vi "SetSomeDataByLabVIEW.vi"() -> ()   [LabVIEW 2020]
panel:
  out "SLM_NewPulseParameters":cluster{"Freq":i32, "PulseMode":u8}
  out "SOMD_Sync":bool
  out "SOMD_NewBurstValues":T1
  out "VIR_NewFanRunning":bool
  out "VUV_NewFanRunning":bool
  out "VIR_NewIntensity":i32
  out "VUV_NewIntensity":i32
  out "VIR_NewFreqDivIdx":i32
  out "VUV_NewFreqDivIdx":i32
  out "VIR_NewTrigSrcIdx":i32
  out "VUV_NewTrigSrcIdx":i32
  out "VUV_NewTriggerLevel":i32
  out "VIR_NewTriggerLevel":i32
  out "IsVIRModule":bool
  out "VUV_VIR_ModuleType":i32
  out "SOM_NewBurstLengthArray":i32[](array[numeric])
  out "SOM_NewOutNSyncEnable":T2 {"OutEnable" format="%08b"; "SyncEnable" format="%08b"}
  out "SOM_NewBurstValues":T3
  out "SOM_NewFreqTrigMode":i32
  out "SLM_NewIntensity":u16
  out "PRI_NewIntensity":u16
  out "PRI_NewWLIdx":i32
  out "PRI_NewOpModeIdx":i32
  out "Lib Version":string
  out "ModTypAbbr":T4
  out "IsSOMDModule":bool
  out "SOM_ModuleType":i32
  out "PRIConst":T5={"bInitialized"=FALSE, "PrimaModuleID"="", "PrimaModuleType"="", "PrimaFWVers"="", "PrimaTemp_min"=15.0, "PrimaTemp_max"=42.0, "PrimaUSBIdx"=-1, "PrimaSlotId"=-1, "PrimaWLCount"=-1, "PrimaWLs"=[0, 0, 0, -1, -1, -1], "PrimaOpModCount"=-1, "PrimaOpModOff"=-1, "PrimaOpModNarrow"=-1, "PrimaOpModBroad"=-1, "PrimaOpModCW"=-1, "PrimaTrSrcCount"=-1, "PrimaTrSrcInt"=-1, "PrimaTrSrcExtNIM"=-1, "PrimaTrSrcExtTTL"=-1, "PrimaTrSrcExtFallling"=-1, "PrimaTrSrcExtRising"=-1} {"PrimaTemp_min" format="%4.1f"; "PrimaTemp_max" format="%4.1f"; "PrimaSlotId" format="%03d"}
  out "SlotNrsFound":T6 {"SOMSlot" format="%03d"; "SLMSlot" format="%03d"; "VUVSlot" format="%03d"; "VIRSlot" format="%03d"; "PRISlot" format="%03d"}
  out "SerNrsFound":T7
  out "ModTypFound":T8
  out "FW Version":string
  out "clLastFWError":T9
  out "cLastErrorPhase":string
  out "cLastErrorText":string
  out "cProductModel":string caption="Product Model"
  out "cDisplay":string
  out "error out":errorcluster
  out "cDescriptor":string caption="Descriptor"
  in  "iPerformRestart":bool caption="Restart"
  out "iModuleCount":i32 caption="Modules"
  out "cSerialNumber":string caption="Serial Number"
  in  "error in (no error)":errorcluster
  in  "iDevIdx":i32 caption="Device Index" min=0 max=7 step=1
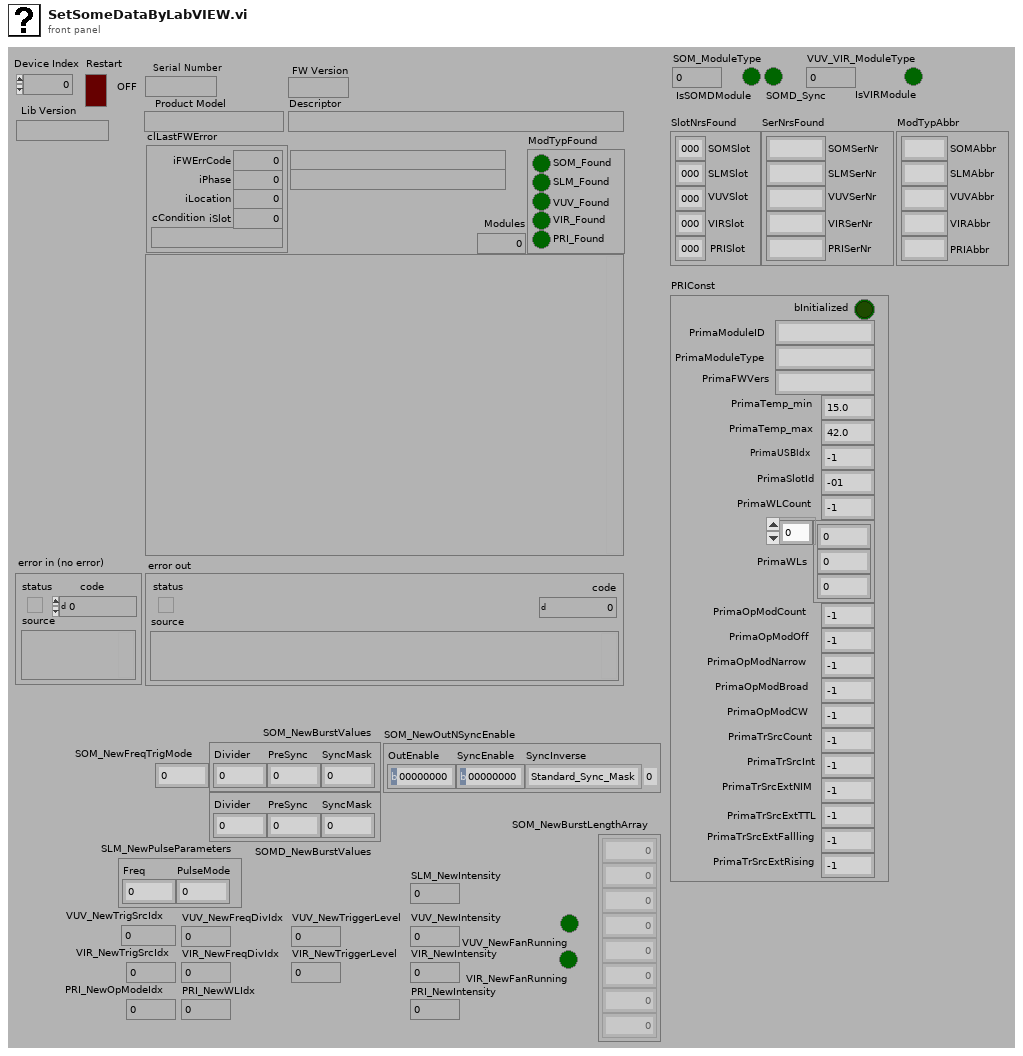
[diagram p1: front panel]
types:
  T1 = cluster{"Divider":u16, "PreSync":u8, "SyncMask":u8}
  T2 = cluster{"OutEnable":u8, "SyncEnable":u8, "SyncInverse":enum8{"Standard_Sync_Mask", "Inverse_Sync_Mask"}}
  T3 = cluster{"Divider":u8, "PreSync":u8, "SyncMask":u8}
  T4 = cluster{"SOMAbbr":string, "SLMAbbr":string, "VUVAbbr":string, "VIRAbbr":string, "PRIAbbr":string}
  T5 = cluster{"bInitialized":bool, "PrimaModuleID":string, "PrimaModuleType":string, "PrimaFWVers":string, "PrimaTemp_min":sgl, "PrimaTemp_max":sgl, "PrimaUSBIdx":i32, "PrimaSlotId":i32, "PrimaWLCount":i32, "PrimaWLs":i32[], "PrimaOpModCount":i32, "PrimaOpModOff":i32, "PrimaOpModNarrow":i32, "PrimaOpModBroad":i32, "PrimaOpModCW":i32, "PrimaTrSrcCount":i32, "PrimaTrSrcInt":i32, "PrimaTrSrcExtNIM":i32, "PrimaTrSrcExtTTL":i32, "PrimaTrSrcExtFallling":i32, "PrimaTrSrcExtRising":i32}
  T6 = cluster{"SOMSlot":i32, "SLMSlot":i32, "VUVSlot":i32, "VIRSlot":i32, "PRISlot":i32}
  T7 = cluster{"SOMSerNr":string, "SLMSerNr":string, "VUVSerNr":string, "VIRSerNr":string, "PRISerNr":string}
  T8 = cluster{"SOM_Found":bool, "SLM_Found":bool, "VUV_Found":bool, "VIR_Found":bool, "PRI_Found":bool}
  T9 = cluster{"iFWErrCode":i32, "iPhase":i32, "iLocation":i32, "iSlot":i32, "cCondition":string}
  T10 = enum16{"open", "replace", "create", "open or create", "replace or create", "replace or create with confirmation"}
  T11 = cluster{"ErrCode":i32, "Error Text":string, "Phase":i32, "Phase Text":string, "Location":i32, "Slot":i32, "Condition":string}
  T12 = cluster{"SlotId":i32, "IsPrimary":u8, "IsBackPlane":u8, "HasUptimeCounter":u8}
  T13 = cluster{"Freq":i32, "PulseMode":u8, "HeadType":i32}
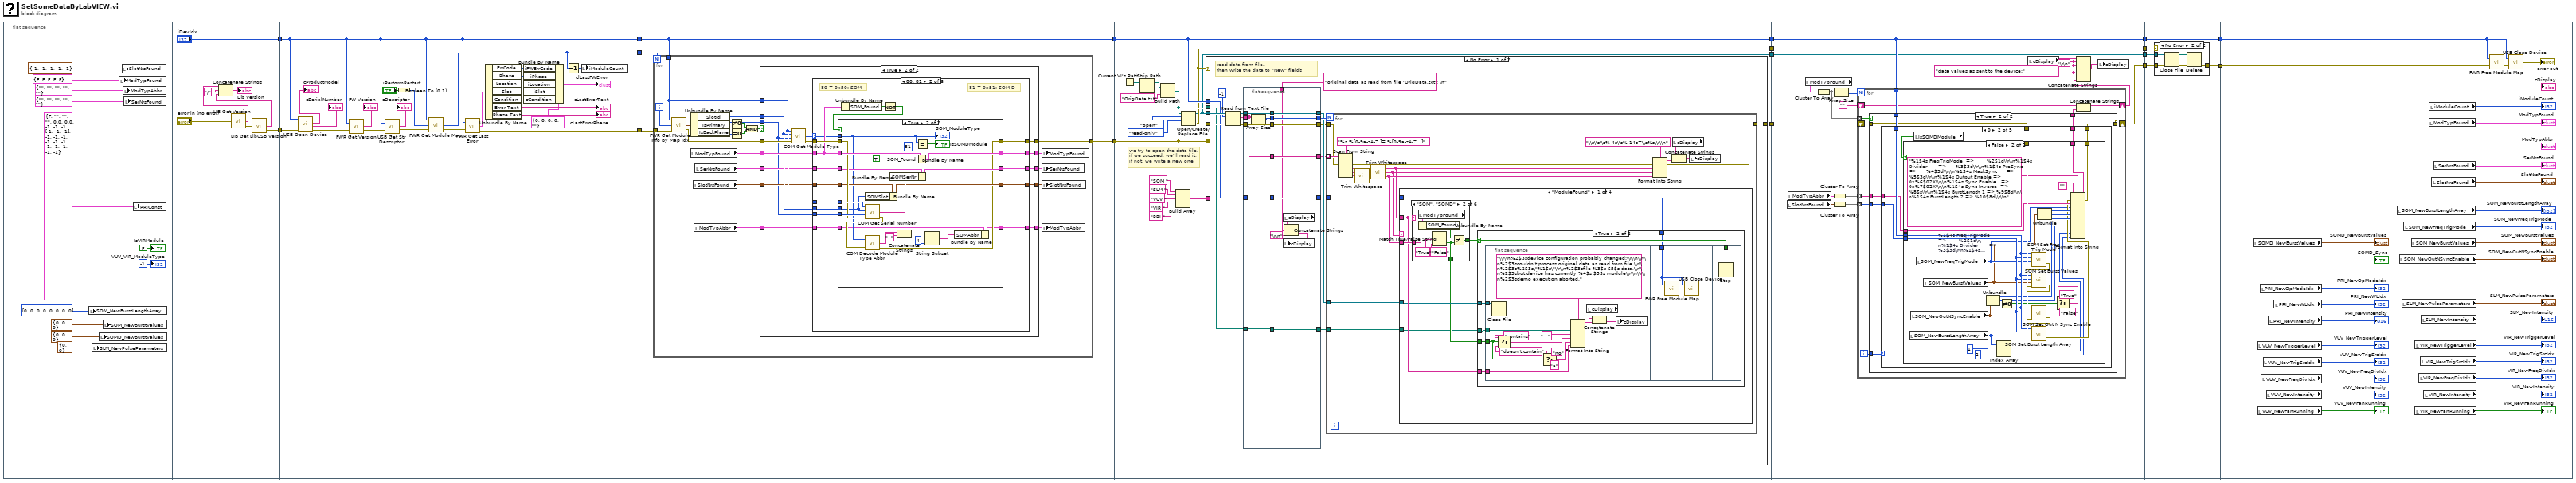
[diagram p0: block diagram]
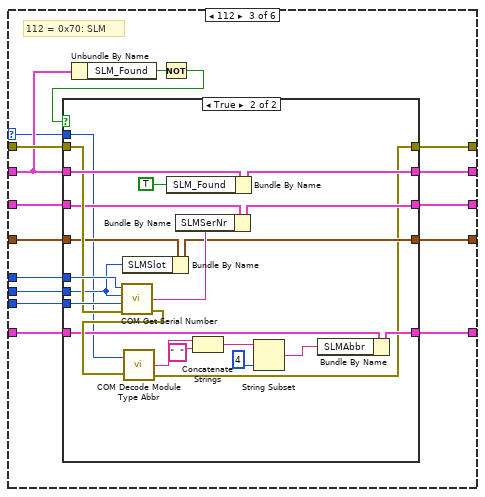
[diagram p5: hidden frame]
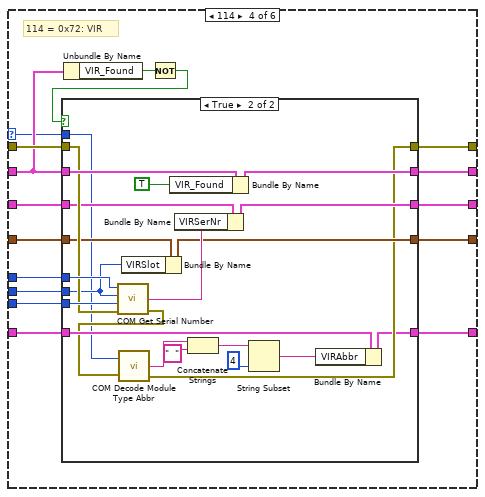
[diagram p7: hidden frame]
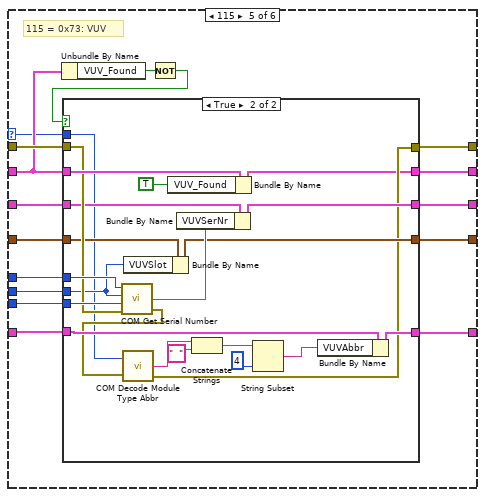
[diagram p9: hidden frame]
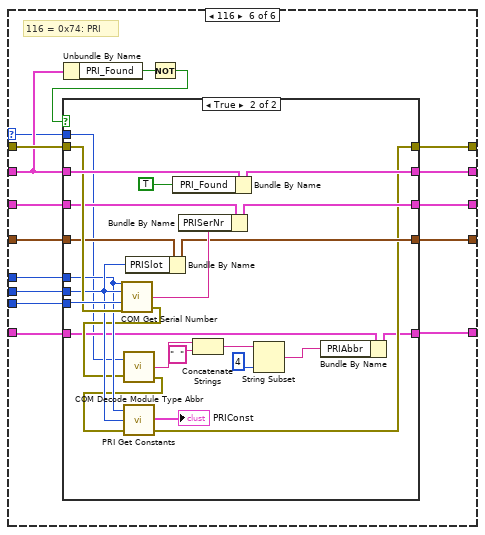
[diagram p11: hidden frame]
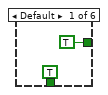
[diagram p14: hidden frame]
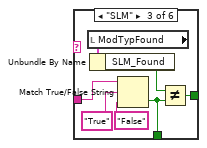
[diagram p15: hidden frame]
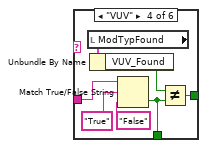
[diagram p16: hidden frame]
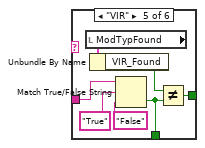
[diagram p17: hidden frame]
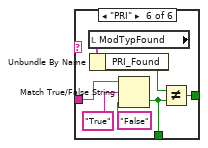
[diagram p18: hidden frame]
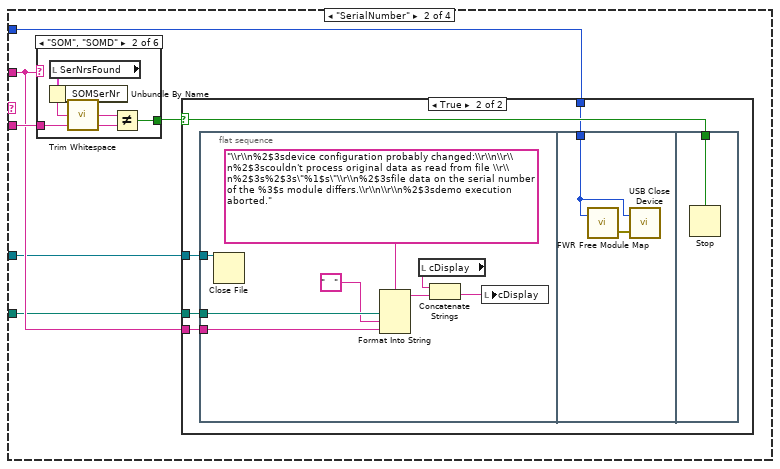
[diagram p19: hidden frame]
diagram:
  n1 = flat-sequence {
    tunnel: ["iDevIdx"] -> w17
    tunnel: [w29] -> w16
    tunnel: w17 -> [w61]
    tunnel: w16 -> [w39]
    tunnel: [w61] -> w15
    tunnel: [w37] -> w14
    tunnel: [w38] -> w13
    tunnel: w15 -> [w62]
    tunnel: w14 -> [w64]
    tunnel: w13 -> [w63]
    tunnel: [w65] -> w12
    tunnel: [w62] -> w11
    tunnel: w12 -> [w334]
    tunnel: w11 -> [w333]
    tunnel: [w333] -> w10
    tunnel: [w332] -> w9
    tunnel: [w331] -> w4
    tunnel: [w330] -> w2
    tunnel: w10 -> [w1031]
    tunnel: w9 -> [w1033]
    tunnel: [w1031] -> w8
    tunnel: [w1032] -> w6
    tunnel: w4 -> [w1027]
    tunnel: [w1027] -> w3
    tunnel: w2 -> [w1026]
    tunnel: [w1026] -> w1
    tunnel: w8 -> [w1206]
    tunnel: [w1206] -> w7
    tunnel: w6 -> [w1203]
    tunnel: [w1202] -> w5
    tunnel: w3 -> [w1205]
    tunnel: w1 -> [w1204]
    tunnel: w7 -> [w1214]
    tunnel: w5 -> [w1213]
    frame #0 {
      n2 = local write "SOM_NewBurstLengthArray"(i32[] [0, 0, 0, 0, 0, 0, 0, 0] ("SOM_NewBurstLengthArray")) -> ()
      n3 = local write "SLM_NewPulseParameters"(cluster{"Freq":i32, "PulseMode":u8} {"Freq"=0, "PulseMode"=0} ("SLM_NewPulseParameters")) -> ()
      n4 = local write "SOMD_NewBurstValues"(T1 {"Divider"=0, "PreSync"=0, "SyncMask"=0} ("SOM_NewBurstValues")) -> ()
      n5 = local write "SOM_NewBurstValues"(T3 {"Divider"=0, "PreSync"=0, "SyncMask"=0} ("SOM_NewBurstValues")) -> ()
      n6 = local write "ModTypFound"(T8 {"SOM_Found"=FALSE, "SLM_Found"=FALSE, "VUV_Found"=FALSE, "VIR_Found"=FALSE, "PRI_Found"=FALSE} ("ModTypFound")) -> ()
      n7 = local write "SlotNrsFound"(T6 {"SOMSlot"=-1, "SLMSlot"=-1, "VUVSlot"=-1, "VIRSlot"=-1, "PRISlot"=-1} ("SlotNrsFound")) -> ()
      n8 = local write "ModTypAbbr"(T4 {"SOMAbbr"="", "SLMAbbr"="", "VUVAbbr"="", "VIRAbbr"="", "PRIAbbr"=""} ("ModTypAbbr")) -> ()
      n9 = local write "SerNrsFound"(T4 {"SOMAbbr"="", "SLMAbbr"="", "VUVAbbr"="", "VIRAbbr"="", "PRIAbbr"=""} ("ModTypAbbr")) -> ()
      n10 = local write "PRIConst"(T5 {"bInitialized"=FALSE, "PrimaModuleID"="", "PrimaModuleType"="", "PrimaFWVers"="", "PrimaTemp_min"=0.0, "PrimaTemp_max"=0.0, "PrimaUSBIdx"=-1, "PrimaSlotId"=-1, "PrimaWLCount"=-1, "PrimaWLs"=[-1, -1, -1], "PrimaOpModCount"=-1, "PrimaOpModOff"=-1, "PrimaOpModNarrow"=-1, "PrimaOpModBroad"=-1, "PrimaOpModCW"=-1, "PrimaTrSrcCount"=-1, "PrimaTrSrcInt"=-1, "PrimaTrSrcExtNIM"=-1, "PrimaTrSrcExtTTL"=-1, "PrimaTrSrcExtFallling"=-1, "PrimaTrSrcExtRising"=-1} ("PRIConst")) -> ()
      "IsVIRModule" <- FALSE ("IsVIRModule")
      "VUV_VIR_ModuleType" <- -1 ("VUV_VIR_ModuleType")
    }
    frame #1 {
      n11 = call "LIB Get Version.vi"("error in (no error)"="error in (no error)") -> ("LibVersion"=w34:string, "error out"=w32:errorcluster)  [unwired: 1 out]
      n12 = call "LIB Get LibUSB Version.vi"("error in (no error)"=w32) -> ("LibUSBVersion"=w33:string, "error out"=w29:errorcluster)  [unwired: 1 out]
      n13 = Concatenate Strings(w34, "/" ("string"), w33) -> (→"Lib Version":string)
    }
    frame #2 {
      n14 = call "USB Open Device.vi"("error in (no error)"=w39, "DevIdx"=w61) -> ("error out"=w57:errorcluster, "SerialNumber"=→"cSerialNumber":string, "ProductModel"=→"cProductModel":string)  [unwired: 2 in, 1 out]
      n15 = call "FWR Get Version.vi"("DevIdx"=w61, "error in (no error)"=w57) -> ("FWVersion"=→"FW Version":string, "error out"=w58:errorcluster)  [unwired: 1 out]
      n16 = call "USB Get Str Descriptor.vi"("DevIdx"=w61, "error in (no error)"=w58) -> ("Descriptor"=→"cDescriptor":string, "error out"=w41:errorcluster)  [unwired: 1 out]
      n17 = Boolean To (0,1)(Boolean="iPerformRestart") -> (0, 1=w55:i16)
      n18 = call "FWR Get Module Map.vi"("error in (no error)"=w41, "PerformRestart"=w55, "DevIdx"=w61) -> ("error out"=w43:errorcluster, "ModuleCount"=w38:i32)  [unwired: 1 out]
      n19 = call "FWR Get Last Error.vi"("DevIdx"=w61, "error in (no error)"=w43) -> ("Last Error"=w54:T11, "error out"=w37:errorcluster)  [unwired: 1 out]
      n20 = Unbundle By Name(w54) -> ("ErrCode"=w46:i32, "Phase"=w47:i32, "Location"=w48:i32, "Slot"=w49:i32, "Condition"=w50:string, "Error Text"=→"cLastErrorText":string, "Phase Text"=→"cLastErrorPhase":string)
      n21 = Bundle By Name(cluster=T9 {"iFWErrCode"=0, "iPhase"=0, "iLocation"=0, "iSlot"=0, "cCondition"=""} ("clLastFWError"), "iFWErrCode"=w46, "iPhase"=w47, "iLocation"=w48, "iSlot"=w49, "cCondition"=w50) -> (→"clLastFWError":T9)
      n22 = Decrement(x=w38) -> (x-1=w60:i32)
      n23 = local write "iModuleCount"(w60) -> ()
    }
    frame #3 {
      n24 = for {
        N: w63 -> [_]
        tunnel: [w75] -> w65
        tunnel: w64 -> [w76]
        tunnel: w62 -> [w78]
        i -> [w84]
        n25 = call "FWR Get Module Info By Map Idx.vi"("error in (no error)"=w76, "MapIdx"=w84, "DevIdx"=w78) -> ("error out"=w74:errorcluster, "FWR Module Info"=w85:T12)  [unwired: 1 out]
        n26 = local read "ModTypFound"() -> (w73:T8)
        n27 = Unbundle By Name(w85) -> ("SlotId"=w79:i32, "IsPrimary"=w77:u8, "IsBackPlane"=w83:u8)
        n28 = local read "SlotNrsFound"() -> (w69:T6)
        n29 = local read "ModTypAbbr"() -> (w67:T4)
        n30 = local read "SerNrsFound"() -> (w71:T7)
        n31 = Not Equal To 0?(x=w77) -> (x != 0?=w81:bool)
        n32 = Equal To 0?(x=w83) -> (x = 0?=w82:bool)
        n33 = And(x=w81, y=w82) -> (x .and. y?=w80:bool)
        n34 = case shown="True" w80 {
          tunnel: w79 -> [_ w98]
          tunnel: w78 -> [_ w99]
          tunnel: w77 -> [_ w91]
          tunnel: w74 -> [w90 w105]
          tunnel: [w90 w103] -> w75
          tunnel: w73 -> [w89 w101]
          tunnel: [w89 w100] -> w72
          tunnel: w71 -> [w88 w97]
          tunnel: [w88 w96] -> w70
          tunnel: w69 -> [w87 w95]
          tunnel: [w87 w94] -> w68
          tunnel: w67 -> [w86 w93]
          tunnel: [w86 w92] -> w66
          frame False {
          }
          frame True {
            n35 = call "COM Get Module Type.vi"("error in (no error)"=w105, "GetPrimary"=w91, "SlotId"=w98, "DevIdx"=w99) -> ("error out"=w104:errorcluster, "ModuleType"=w102:i32)  [unwired: 1 out]
            n36 = case shown="80, 81" w102 {
              selector: w102 -> [_ w113 w156 w199 w242 w285]
              tunnel: w104 -> [w109 w125 w170 w213 w256 w299]
              tunnel: [w109 w124 w169 w212 w255 w298] -> w103
              tunnel: w101 -> [w110 w123 w168 w211 w254 w297]
              tunnel: [w110 w126 w171 w214 w257 w300] -> w100
              tunnel: w99 -> [_ w120 w165 w208 w251 w294]
              tunnel: w98 -> [_ w119 w164 w207 w250 w293]
              tunnel: w91 -> [_ w118 w163 w206 w249 w292]
              tunnel: w97 -> [w108 w117 w162 w205 w248 w291]
              tunnel: [w108 w116 w161 w204 w247 w290] -> w96
              tunnel: w95 -> [w107 w115 w160 w203 w246 w289]
              tunnel: [w107 w114 w159 w202 w245 w288] -> w94
              tunnel: w93 -> [w106 w112 w158 w201 w244 w287]
              tunnel: [w106 w111 w157 w200 w243 w286] -> w92
              frame -1, Default {
              }
              frame 80, 81 {
                # "81 = 0x51: SOM-D"
                # "80 = 0x50: SOM"
                n37 = Unbundle By Name(w123) -> ("SOM_Found"=w122:bool)
                n38 = Not(x=w122) -> (.not. x?=w121:bool)
                n39 = case shown="True" w121 {
                  tunnel: w123 -> [w130 w155]
                  tunnel: [w130 w154] -> w126
                  tunnel: w125 -> [w131 w150]
                  tunnel: [w131 w139] -> w124
                  tunnel: w120 -> [_ w152]
                  tunnel: w119 -> [_ w145]
                  tunnel: w118 -> [_ w151]
                  tunnel: w117 -> [w129 w149]
                  tunnel: [w129 w148] -> w116
                  tunnel: w115 -> [w128 w146]
                  tunnel: [w128 w144] -> w114
                  tunnel: w113 -> [_ w140]
                  tunnel: w112 -> [w127 w138]
                  tunnel: [w127 w137] -> w111
                  frame False {
                  }
                  frame True {
                    n40 = Bundle By Name(cluster=w146, "SOMSlot"=w145) -> (w144:T6)
                    n41 = call "COM Get Serial Number.vi"("error in (no error)"=w150, "GetPrimary"=w151, "SlotId"=w145, "DevIdx"=w152) -> ("error out"=w141:errorcluster, "SerialNumber"=w147:string)  [unwired: 1 out]
                    n42 = call "COM Decode Module Type Abbr.vi"("ModuleType"=w140, "error in (no error)"=w141) -> ("ModulTypeAbbr"=w136:string, "error out"=w139:errorcluster)  [unwired: 1 out]
                    n43 = Bundle By Name(cluster=w155, "SOM_Found"=TRUE ("PRI_Found")) -> (w154:T8)
                    n44 = Bundle By Name(cluster=w149, "SOMSerNr"=w147) -> (w148:T7)
                    n45 = Concatenate Strings(w136, "  ") -> (w134:string)
                    n46 = Equal?(x=w140, y=81) -> (x = y?=→"IsSOMDModule":bool)
                    n47 = String Subset(string=w134, length (rest)=4 ("length (rest)")) -> (substring=w132:string)  [unwired: 1 in]
                    n48 = Bundle By Name(cluster=w138, "SOMAbbr"=w132) -> (w137:T4)
                    "SOM_ModuleType" <- w140
                  }
                }
              }
              frame 112 {
                # "112 = 0x70: SLM"
                n49 = Unbundle By Name(w168) -> ("SLM_Found"=w167:bool)
                n50 = Not(x=w167) -> (.not. x?=w166:bool)
                n51 = case shown="True" w166 {
                  tunnel: w168 -> [w175 w198]
                  tunnel: [w175 w197] -> w171
                  tunnel: w170 -> [w176 w193]
                  tunnel: [w176 w179] -> w169
                  tunnel: w165 -> [_ w195]
                  tunnel: w164 -> [_ w188]
                  tunnel: w163 -> [_ w194]
                  tunnel: w162 -> [w174 w192]
                  tunnel: [w174 w191] -> w161
                  tunnel: w160 -> [w173 w189]
                  tunnel: [w173 w187] -> w159
                  tunnel: w158 -> [w172 w178]
                  tunnel: [w172 w181] -> w157
                  tunnel: w156 -> [_ w177]
                  frame False {
                  }
                  frame True {
                    n52 = call "COM Get Serial Number.vi"("error in (no error)"=w193, "GetPrimary"=w194, "SlotId"=w188, "DevIdx"=w195) -> ("error out"=w180:errorcluster, "SerialNumber"=w190:string)  [unwired: 1 out]
                    n53 = Bundle By Name(cluster=w189, "SLMSlot"=w188) -> (w187:T6)
                    n54 = call "COM Decode Module Type Abbr.vi"("ModuleType"=w177, "error in (no error)"=w180) -> ("ModulTypeAbbr"=w186:string, "error out"=w179:errorcluster)  [unwired: 1 out]
                    n55 = Bundle By Name(cluster=w198, "SLM_Found"=TRUE ("PRI_Found")) -> (w197:T8)
                    n56 = Bundle By Name(cluster=w192, "SLMSerNr"=w190) -> (w191:T7)
                    n57 = Concatenate Strings(w186, "  ") -> (w184:string)
                    n58 = String Subset(string=w184, length (rest)=4 ("length (rest)")) -> (substring=w182:string)  [unwired: 1 in]
                    n59 = Bundle By Name(cluster=w178, "SLMAbbr"=w182) -> (w181:T4)
                  }
                }
              }
              frame 114 {
                # "114 = 0x72: VIR"
                n60 = Unbundle By Name(w211) -> ("VIR_Found"=w210:bool)
                n61 = Not(x=w210) -> (.not. x?=w209:bool)
                n62 = case shown="True" w209 {
                  tunnel: w211 -> [w218 w241]
                  tunnel: [w218 w240] -> w214
                  tunnel: w213 -> [w219 w236]
                  tunnel: [w219 w222] -> w212
                  tunnel: w208 -> [_ w238]
                  tunnel: w207 -> [_ w231]
                  tunnel: w206 -> [_ w237]
                  tunnel: w205 -> [w217 w235]
                  tunnel: [w217 w234] -> w204
                  tunnel: w203 -> [w216 w232]
                  tunnel: [w216 w230] -> w202
                  tunnel: w201 -> [w215 w224]
                  tunnel: [w215 w221] -> w200
                  tunnel: w199 -> [_ w220]
                  frame False {
                  }
                  frame True {
                    n63 = call "COM Get Serial Number.vi"("error in (no error)"=w236, "GetPrimary"=w237, "SlotId"=w231, "DevIdx"=w238) -> ("error out"=w223:errorcluster, "SerialNumber"=w233:string)  [unwired: 1 out]
                    n64 = call "COM Decode Module Type Abbr.vi"("ModuleType"=w220, "error in (no error)"=w223) -> ("ModulTypeAbbr"=w229:string, "error out"=w222:errorcluster)  [unwired: 1 out]
                    n65 = Bundle By Name(cluster=w232, "VIRSlot"=w231) -> (w230:T6)
                    n66 = Bundle By Name(cluster=w241, "VIR_Found"=TRUE ("PRI_Found")) -> (w240:T8)
                    n67 = Bundle By Name(cluster=w235, "VIRSerNr"=w233) -> (w234:T7)
                    n68 = Concatenate Strings(w229, "  ") -> (w227:string)
                    n69 = String Subset(string=w227, length (rest)=4 ("length (rest)")) -> (substring=w225:string)  [unwired: 1 in]
                    n70 = Bundle By Name(cluster=w224, "VIRAbbr"=w225) -> (w221:T4)
                  }
                }
              }
              frame 115 {
                # "115 = 0x73: VUV"
                n71 = Unbundle By Name(w254) -> ("VUV_Found"=w253:bool)
                n72 = Not(x=w253) -> (.not. x?=w252:bool)
                n73 = case shown="True" w252 {
                  tunnel: w254 -> [w261 w284]
                  tunnel: [w261 w263] -> w257
                  tunnel: w256 -> [w262 w280]
                  tunnel: [w262 w265] -> w255
                  tunnel: w251 -> [_ w282]
                  tunnel: w250 -> [_ w275]
                  tunnel: w249 -> [_ w281]
                  tunnel: w248 -> [w260 w279]
                  tunnel: [w260 w278] -> w247
                  tunnel: w246 -> [w259 w276]
                  tunnel: [w259 w274] -> w245
                  tunnel: w244 -> [w258 w268]
                  tunnel: [w258 w267] -> w243
                  tunnel: w242 -> [_ w264]
                  frame False {
                  }
                  frame True {
                    n74 = call "COM Get Serial Number.vi"("error in (no error)"=w280, "GetPrimary"=w281, "SlotId"=w275, "DevIdx"=w282) -> ("error out"=w266:errorcluster, "SerialNumber"=w277:string)  [unwired: 1 out]
                    n75 = call "COM Decode Module Type Abbr.vi"("ModuleType"=w264, "error in (no error)"=w266) -> ("ModulTypeAbbr"=w273:string, "error out"=w265:errorcluster)  [unwired: 1 out]
                    n76 = Bundle By Name(cluster=w276, "VUVSlot"=w275) -> (w274:T6)
                    n77 = Bundle By Name(cluster=w284, "VUV_Found"=TRUE ("PRI_Found")) -> (w263:T8)
                    n78 = Bundle By Name(cluster=w279, "VUVSerNr"=w277) -> (w278:T7)
                    n79 = Concatenate Strings(w273, "  ") -> (w271:string)
                    n80 = String Subset(string=w271, length (rest)=4 ("length (rest)")) -> (substring=w269:string)  [unwired: 1 in]
                    n81 = Bundle By Name(cluster=w268, "VUVAbbr"=w269) -> (w267:T4)
                  }
                }
              }
              frame 116 {
                # "116 = 0x74: PRI"
                n82 = Unbundle By Name(w297) -> ("PRI_Found"=w296:bool)
                n83 = Not(x=w296) -> (.not. x?=w295:bool)
                n84 = case shown="True" w295 {
                  tunnel: w297 -> [w304 w329]
                  tunnel: [w304 w328] -> w300
                  tunnel: w299 -> [w305 w325]
                  tunnel: [w305 w316] -> w298
                  tunnel: w294 -> [_ w318]
                  tunnel: w293 -> [_ w319]
                  tunnel: w292 -> [_ w326]
                  tunnel: w291 -> [w303 w324]
                  tunnel: [w303 w323] -> w290
                  tunnel: w289 -> [w302 w321]
                  tunnel: [w302 w320] -> w288
                  tunnel: w287 -> [w301 w308]
                  tunnel: [w301 w307] -> w286
                  tunnel: w285 -> [_ w306]
                  frame False {
                  }
                  frame True {
                    n85 = call "COM Get Serial Number.vi"("error in (no error)"=w325, "GetPrimary"=w326, "SlotId"=w319, "DevIdx"=w318) -> ("error out"=w310:errorcluster, "SerialNumber"=w322:string)  [unwired: 1 out]
                    n86 = call "COM Decode Module Type Abbr.vi"("ModuleType"=w306, "error in (no error)"=w310) -> ("ModulTypeAbbr"=w315:string, "error out"=w309:errorcluster)  [unwired: 1 out]
                    n87 = call "PRI Get Constants.vi"("error in (no error)"=w309, "SlotId"=w319, "DevIdx"=w318) -> ("error out"=w316:errorcluster, "PRIConst"=→"PRIConst":T5)  [unwired: 1 out]
                    n88 = Bundle By Name(cluster=w321, "PRISlot"=w319) -> (w320:T6)
                    n89 = Bundle By Name(cluster=w329, "PRI_Found"=TRUE) -> (w328:T8)
                    n90 = Bundle By Name(cluster=w324, "PRISerNr"=w322) -> (w323:T7)
                    n91 = Concatenate Strings(w315, "  ") -> (w313:string)
                    n92 = String Subset(string=w313, length (rest)=4 ("length (rest)")) -> (substring=w311:string)  [unwired: 1 in]
                    n93 = Bundle By Name(cluster=w308, "PRIAbbr"=w311) -> (w307:T4)
                  }
                }
              }
            }
          }
        }
        n94 = local write "ModTypFound"(w72) -> ()
        n95 = local write "SerNrsFound"(w70) -> ()
        n96 = local write "SlotNrsFound"(w68) -> ()
        n97 = local write "ModTypAbbr"(w66) -> ()
      }
    }
    frame #4 {
      # "we try to open the data file.\nif we succeed, we'll read it,\nif not, we write a new one"
      n98 = Current VI's Path() -> (path=w344:path)
      n99 = Strip Path(path=w344) -> (stripped path=w343:path)  [unwired: 1 out]
      n100 = Build Path(base path=w343, name or relative path="OrigData.txt") -> (appended path=w345:path)
      n101 = Build Array("SOM " ("element"), "SLM " ("element"), "VUV " ("element"), "VIR " ("element"), "PRI " ("element")) -> (w346:string[])
      n102 = Open/Create/Replace File(file path (use dialog)=w345, error in=w334, operation (0:open)=T10."open", access (0:read/write)=enum16{"read/write", "read-only", "write-only"}."read-only") -> (refnum out=w330:refnum<file>, error out=w331:errorcluster)  [unwired: 2 in, 1 out]
      n103 = case shown="No Error" w331 {
        tunnel: w330 -> [w368 _]
        tunnel: w345 -> [w355 w756]
        tunnel: w333 -> [w357 w755]
        tunnel: w334 -> [_ w757]
        tunnel: [w364 w752] -> w332
        tunnel: w331 -> [w366 w753]
        tunnel: w346 -> [_ w751]
        frame No Error {
          # "read data from file, \nthen write the data to \"New\" fields"
          n104 = Read from Text File(file (use dialog)=w368, count=-1, error in=w366) -> (refnum out=w361:refnum<file>, text=w363:string[], error out=w360:errorcluster)  [unwired: 1 in, 1 out]
          n105 = flat-sequence {
            tunnel: w363 -> [w371]
            tunnel: w361 -> [w373]
            tunnel: w360 -> [w372]
            tunnel: w357 -> [w370]
            tunnel: w355 -> [w369]
            tunnel: [w374] -> w353
            tunnel: [w373] -> w352
            tunnel: [w372] -> w351
            tunnel: [w371] -> w350
            tunnel: [w370] -> w349
            tunnel: [w369] -> w348
            tunnel: [w379] -> w354
            tunnel: [w380] -> w356
            tunnel: [w381] -> w358
            tunnel: [w382] -> w359
            tunnel: [w383] -> w362
            tunnel: [w384] -> w365
            tunnel: w353 -> [w384]
            tunnel: w352 -> [w383]
            tunnel: w351 -> [w382]
            tunnel: w350 -> [w381]
            tunnel: w349 -> [w380]
            tunnel: w348 -> [w379]
            tunnel: "original data as read from file 'OrigData.txt': \n" -> [w376]
            frame #0 {
              n106 = Array Size(array=w371) -> (size(s)=w374:i32)
            }
            frame #1 {
              n107 = local read "cDisplay"() -> (w377:string)
              n108 = Concatenate Strings(w377, w376, "\r\n") -> (w378:string)
              n109 = local write "cDisplay"(w378) -> ()
            }
          }
          n110 = for {
            N: w365 -> [_]
            tunnel: [w385] -> w364
            tunnel: w359 -> [w387]
            tunnel: w358 -> [w401] mode=indexing
            tunnel: w362 -> [w390]
            tunnel: w354 -> [w389]
            tunnel: w356 -> [w388]
            n111 = Scan From String(format string="%s %[0-9a-zA-Z ]= %[0-9a-zA-Z., ]", input string=w401, error in=w387) -> (error out=w386:errorcluster, output 1=w394:string, output 2=w395:string, output 3=w393:string)  [unwired: 4 in, 2 out]
            n112 = call <vilib>:"Trim Whitespace.vi"("string"=w393) -> ("trimmed string"=w392:string)  [unwired: 1 in]
            n113 = call <vilib>:"Trim Whitespace.vi"("string"=w395) -> ("trimmed string"=w391:string)  [unwired: 1 in]
            n114 = case shown="\"ModuleFound\"" w391 {
              selector: w391 -> [_ _ _ w567]
              tunnel: w394 -> [w406 w474 w521 w568]
              tunnel: w392 -> [w408 w475 w523 w566]
              tunnel: w390 -> [w405 w472 w520 _]
              tunnel: w389 -> [w402 w473 w519 _]
              tunnel: w388 -> [w403 w471 w518 _]
              frame "ModuleFound" {
                n115 = case shown="\"SOM\", \"SOMD\"" w406 {
                  tunnel: w408 -> [_ w439 w446 w453 w460 w467]
                  tunnel: [TRUE w436 w443 w450 w457 w464] -> w407
                  tunnel: [TRUE ("selection") w435 w442 w449 w456 w463] -> w404
                  frame Default {
                  }
                  frame "SOM", "SOMD" {
                    n116 = local read "ModTypFound"() -> (w441:T8)
                    n117 = Unbundle By Name(w441) -> ("SOM_Found"=w440:bool)
                    n118 = Match True/False String(2:"False", 3:"True", 4:w439) -> (0:w435:bool)  [unwired: 1 out]
                    n119 = Not Equal?(x=w440, y=w435) -> (x != y?=w436:bool)
                  }
                  frame "SLM" {
                    n120 = local read "ModTypFound"() -> (w448:T8)
                    n121 = Unbundle By Name(w448) -> ("SLM_Found"=w447:bool)
                    n122 = Match True/False String(2:"False", 3:"True", 4:w446) -> (0:w442:bool)  [unwired: 1 out]
                    n123 = Not Equal?(x=w447, y=w442) -> (x != y?=w443:bool)
                  }
                  frame "VUV" {
                    n124 = local read "ModTypFound"() -> (w455:T8)
                    n125 = Unbundle By Name(w455) -> ("VUV_Found"=w454:bool)
                    n126 = Match True/False String(2:"False", 3:"True", 4:w453) -> (0:w449:bool)  [unwired: 1 out]
                    n127 = Not Equal?(x=w454, y=w449) -> (x != y?=w450:bool)
                  }
                  frame "VIR" {
                    n128 = local read "ModTypFound"() -> (w462:T8)
                    n129 = Unbundle By Name(w462) -> ("VIR_Found"=w461:bool)
                    n130 = Match True/False String(2:"False", 3:"True", 4:w460) -> (0:w456:bool)  [unwired: 1 out]
                    n131 = Not Equal?(x=w461, y=w456) -> (x != y?=w457:bool)
                  }
                  frame "PRI" {
                    n132 = local read "ModTypFound"() -> (w469:T8)
                    n133 = Unbundle By Name(w469) -> ("PRI_Found"=w468:bool)
                    n134 = Match True/False String(2:"False", 3:"True", 4:w467) -> (0:w463:bool)  [unwired: 1 out]
                    n135 = Not Equal?(x=w468, y=w463) -> (x != y?=w464:bool)
                  }
                }
                n136 = case shown="True" w407 {
                  selector: w407 -> [_ w413]
                  tunnel: w405 -> [_ w414]
                  tunnel: w404 -> [_ w412]
                  tunnel: w402 -> [_ w411]
                  tunnel: w403 -> [_ w410]
                  tunnel: w406 -> [_ w409]
                  frame False {
                  }
                  frame True {
                    n137 = flat-sequence {
                      tunnel: w414 -> [w427]
                      tunnel: w412 -> [w421]
                      tunnel: w411 -> [w424]
                      tunnel: w409 -> [w415]
                      tunnel: w410 -> [w431]
                      tunnel: w413 -> [w432]
                      frame #0 {
                        n138 = Close File(refnum=w427) -> ()  [unwired: 1 in, 2 out]
                        n139 = Select(t="contains", s=w421, f="doesn't contain") -> (s? t:f=w417:string)
                        n140 = Select(t="no", s=w421, f="a") -> (s? t:f=w418:string)
                        n141 = Format Into String(format string="\\r\\n%2$3sdevice configuration probably changed:\\r\\n\\r\\n%2$3scouldn't process original data as read from file \\r\\n%2$3s%2$3s\"%1$s\"\\r\\n%2$3sfile %3$s $5$s data,\\r\\n%2$3sbut device has currently %4$s $5$s module\\r\\n\\r\\n%2$3sdemo execution aborted." ("string"), w424, "   " ("input 2"), w417, w418, w415) -> (resulting string=w426:string)  [unwired: 2 in, 1 out]
                        n142 = local read "cDisplay"() -> (w428:string)
                        n143 = Concatenate Strings(w428, w426) -> (w429:string)
                        n144 = local write "cDisplay"(w429) -> ()
                      }
                      frame #1 {
                        n145 = call "FWR Free Module Map.vi"("DevIdx"=w431) -> ("error out"=w430:errorcluster)  [unwired: 1 in, 1 out]
                        n146 = call "USB Close Device.vi"("error in (no error)"=w430, "DevIdx"=w431) -> ()  [unwired: 1 out]
                      }
                      frame #2 {
                        n147 = Stop(stop? (T)=w432) -> ()
                      }
                    }
                  }
                }
              }
              frame "SerialNumber" {
                n148 = case shown="\"SOM\", \"SOMD\"" w474 {
                  tunnel: w475 -> [_ w496 w501 w506 w511 w516]
                  tunnel: [TRUE w493 w498 w503 w508 w513] -> w470
                  frame Default {
                  }
                  frame "SOM", "SOMD" {
                    n149 = local read "SerNrsFound"() -> (w497:T7)
                    n150 = Unbundle By Name(w497) -> ("SOMSerNr"=w495:string)
                    n151 = call <vilib>:"Trim Whitespace.vi"("string"=w495) -> ("trimmed string"=w494:string)  [unwired: 1 in]
                    n152 = Not Equal?(x=w494, y=w496) -> (x != y?=w493:bool)
                  }
                  frame "SLM" {
                    n153 = local read "SerNrsFound"() -> (w502:T7)
                    n154 = Unbundle By Name(w502) -> ("SLMSerNr"=w500:string)
                    n155 = call <vilib>:"Trim Whitespace.vi"("string"=w500) -> ("trimmed string"=w499:string)  [unwired: 1 in]
                    n156 = Not Equal?(x=w499, y=w501) -> (x != y?=w498:bool)
                  }
                  frame "VUV" {
                    n157 = local read "SerNrsFound"() -> (w507:T7)
                    n158 = Unbundle By Name(w507) -> ("VUVSerNr"=w505:string)
                    n159 = call <vilib>:"Trim Whitespace.vi"("string"=w505) -> ("trimmed string"=w504:string)  [unwired: 1 in]
                    n160 = Not Equal?(x=w504, y=w506) -> (x != y?=w503:bool)
                  }
                  frame "VIR" {
                    n161 = local read "SerNrsFound"() -> (w512:T7)
                    n162 = Unbundle By Name(w512) -> ("VIRSerNr"=w510:string)
                    n163 = call <vilib>:"Trim Whitespace.vi"("string"=w510) -> ("trimmed string"=w509:string)  [unwired: 1 in]
                    n164 = Not Equal?(x=w509, y=w511) -> (x != y?=w508:bool)
                  }
                  frame "PRI" {
                    n165 = local read "SerNrsFound"() -> (w517:T7)
                    n166 = Unbundle By Name(w517) -> ("PRISerNr"=w515:string)
                    n167 = call <vilib>:"Trim Whitespace.vi"("string"=w515) -> ("trimmed string"=w514:string)  [unwired: 1 in]
                    n168 = Not Equal?(x=w514, y=w516) -> (x != y?=w513:bool)
                  }
                }
                n169 = case shown="True" w470 {
                  selector: w470 -> [_ w479]
                  tunnel: w472 -> [_ w480]
                  tunnel: w473 -> [_ w478]
                  tunnel: w471 -> [_ w477]
                  tunnel: w474 -> [_ w476]
                  frame False {
                  }
                  frame True {
                    n170 = flat-sequence {
                      tunnel: w480 -> [w486]
                      tunnel: w478 -> [w483]
                      tunnel: w476 -> [w481]
                      tunnel: w477 -> [w490]
                      tunnel: w479 -> [w491]
                      frame #0 {
                        n171 = Close File(refnum=w486) -> ()  [unwired: 1 in, 2 out]
                        n172 = Format Into String(format string="\\r\\n%2$3sdevice configuration probably changed:\\r\\n\\r\\n%2$3scouldn't process original data as read from file \\r\\n%2$3s%2$3s\"%1$s\"\\r\\n%2$3sfile data on the serial number of the %3$s module differs.\\r\\n\\r\\n%2$3sdemo execution aborted." ("string"), w483, "   " ("input 2"), w481) -> (resulting string=w485:string)  [unwired: 2 in, 1 out]
                        n173 = local read "cDisplay"() -> (w487:string)
                        n174 = Concatenate Strings(w487, w485) -> (w488:string)
                        n175 = local write "cDisplay"(w488) -> ()
                      }
                      frame #1 {
                        n176 = call "FWR Free Module Map.vi"("DevIdx"=w490) -> ("error out"=w489:errorcluster)  [unwired: 1 in, 1 out]
                        n177 = call "USB Close Device.vi"("error in (no error)"=w489, "DevIdx"=w490) -> ()  [unwired: 1 out]
                      }
                      frame #2 {
                        n178 = Stop(stop? (T)=w491) -> ()
                      }
                    }
                  }
                }
              }
              frame "SlotID" {
                n179 = case shown="\"PRI\"" w521 {
                  tunnel: w523 -> [_ w543 w548 w553 w558 w563]
                  tunnel: [TRUE w541 w546 w551 w556 w561] -> w522
                  frame Default {
                  }
                  frame "SOM", "SOMD" {
                    n180 = local read "SlotNrsFound"() -> (w545:T6)
                    n181 = Unbundle By Name(w545) -> ("SOMSlot"=w544:i32)
                    n182 = Decimal String To Number(string=w543) -> (number=w542:i32)  [unwired: 2 in, 1 out]
                    n183 = Not Equal?(x=w544, y=w542) -> (x != y?=w541:bool)
                  }
                  frame "SLM" {
                    n184 = local read "SlotNrsFound"() -> (w550:T6)
                    n185 = Unbundle By Name(w550) -> ("SLMSlot"=w549:i32)
                    n186 = Decimal String To Number(string=w548) -> (number=w547:i32)  [unwired: 2 in, 1 out]
                    n187 = Not Equal?(x=w549, y=w547) -> (x != y?=w546:bool)
                  }
                  frame "VUV" {
                    n188 = local read "SlotNrsFound"() -> (w555:T6)
                    n189 = Unbundle By Name(w555) -> ("VUVSlot"=w554:i32)
                    n190 = Decimal String To Number(string=w553) -> (number=w552:i32)  [unwired: 2 in, 1 out]
                    n191 = Not Equal?(x=w554, y=w552) -> (x != y?=w551:bool)
                  }
                  frame "VIR" {
                    n192 = local read "SlotNrsFound"() -> (w560:T6)
                    n193 = Unbundle By Name(w560) -> ("VIRSlot"=w559:i32)
                    n194 = Decimal String To Number(string=w558) -> (number=w557:i32)  [unwired: 2 in, 1 out]
                    n195 = Not Equal?(x=w559, y=w557) -> (x != y?=w556:bool)
                  }
                  frame "PRI" {
                    n196 = local read "SlotNrsFound"() -> (w565:T6)
                    n197 = Unbundle By Name(w565) -> ("PRISlot"=w564:i32)
                    n198 = Decimal String To Number(string=w563) -> (number=w562:i32)  [unwired: 2 in, 1 out]
                    n199 = Not Equal?(x=w564, y=w562) -> (x != y?=w561:bool)
                  }
                }
                n200 = case shown="True" w522 {
                  selector: w522 -> [_ w527]
                  tunnel: w520 -> [_ w528]
                  tunnel: w519 -> [_ w526]
                  tunnel: w518 -> [_ w525]
                  tunnel: w521 -> [_ w524]
                  tunnel: w522 -> [_ _]
                  frame False {
                  }
                  frame True {
                    n201 = flat-sequence {
                      tunnel: w528 -> [w534]
                      tunnel: w526 -> [w531]
                      tunnel: w524 -> [w529]
                      tunnel: w525 -> [w538]
                      tunnel: w527 -> [w539]
                      frame #0 {
                        n202 = Close File(refnum=w534) -> ()  [unwired: 1 in, 2 out]
                        n203 = Format Into String(format string="\\r\\n%2$3sdevice configuration probably changed:\\r\\n\\r\\n%2$3scouldn't process original data as read from file \\r\\n%2$3s%2$3s\"%1$s\"\\r\\n%2$3sfile data on the slot number of the %3$s module differs.\\r\\n\\r\\n%2$3sdemo execution aborted." ("string"), w531, "   " ("input 2"), w529) -> (resulting string=w533:string)  [unwired: 2 in, 1 out]
                        n204 = local read "cDisplay"() -> (w535:string)
                        n205 = Concatenate Strings(w535, w533) -> (w536:string)
                        n206 = local write "cDisplay"(w536) -> ()
                      }
                      frame #1 {
                        n207 = call "FWR Free Module Map.vi"("DevIdx"=w538) -> ("error out"=w537:errorcluster)  [unwired: 1 in, 1 out]
                        n208 = call "USB Close Device.vi"("error in (no error)"=w537, "DevIdx"=w538) -> ()  [unwired: 1 out]
                      }
                      frame #2 {
                        n209 = Stop(stop? (T)=w539) -> ()
                      }
                    }
                  }
                }
              }
              frame Default {
                n210 = case shown="\"VIR\", \"VUV\"" w568 {
                  selector: w568 -> [_ _ _ _ w705 _]
                  tunnel: w567 -> [_ w570 w627 w684 w707 w740]
                  tunnel: w566 -> [_ w569 w626 w683 w706 w739]
                  frame Default {
                  }
                  frame "SOM" {
                    n211 = case shown="\"Divider\", \"MaskSync\", \"PreSync\"" w570 {
                      selector: w570 -> [_ w576 w594 w620 _]
                      tunnel: w569 -> [w572 w575 w593 w619 _]
                      frame "FreqTrigMode" {
                        n212 = Decimal String To Number(string=w572) -> (number=w571:i32)  [unwired: 2 in, 1 out]
                        n213 = local write "SOM_NewFreqTrigMode"(w571) -> ()
                      }
                      frame "Divider", "MaskSync", "PreSync" {
                        n214 = local read "SOM_NewBurstValues"() -> (w573:T3)
                        n215 = case shown="\"Divider\"" w576 {
                          tunnel: w575 -> [_ w582 w587 w592]
                          tunnel: [w577 w581 w586 w591] -> w574
                          tunnel: w573 -> [w577 w580 w585 w590]
                          frame Default {
                          }
                          frame "Divider" {
                            n216 = Decimal String To Number(string=w582, default (0L)=u8 0 ("default (0 I32)")) -> (number=w579:u8)  [unwired: 1 in, 1 out]
                            n217 = Bundle By Name(cluster=w580, "Divider"=w579) -> (w581:T3)
                          }
                          frame "PreSync" {
                            n218 = Decimal String To Number(string=w587, default (0L)=u8 0 ("default (0 I32)")) -> (number=w584:u8)  [unwired: 1 in, 1 out]
                            n219 = Bundle By Name(cluster=w585, "PreSync"=w584) -> (w586:T3)
                          }
                          frame "MaskSync" {
                            n220 = Decimal String To Number(string=w592, default (0L)=u8 0 ("default (0 I32)")) -> (number=w589:u8)  [unwired: 1 in, 1 out]
                            n221 = Bundle By Name(cluster=w590, "SyncMask"=w589) -> (w591:T3)
                          }
                        }
                        n222 = local write "SOM_NewBurstValues"(w574) -> ()
                      }
                      frame "Output Enable", "Sync Enable", "Sync Inverse" {
                        n223 = local read "SOM_NewOutNSyncEnable"() -> (w595:T2)
                        n224 = case shown="\"Sync Inverse\"" w594 {
                          tunnel: [w597 w603 w609 w617] -> w596
                          tunnel: w595 -> [w597 w602 w608 w616]
                          tunnel: w593 -> [_ w601 w607 w613]
                          frame Default {
                          }
                          frame "Output Enable" {
                            n225 = Hexadecimal String To Number(string=w601, offset=2, default (0uL)=u8 0 ("default (0 U32)")) -> (number=w598:u8)  [unwired: 1 out]
                            n226 = Bundle By Name(cluster=w602, "OutEnable"=w598) -> (w603:T2)
                          }
                          frame "Sync Enable" {
                            n227 = Hexadecimal String To Number(string=w607, offset=2, default (0uL)=u8 0 ("default (0 U32)")) -> (number=w604:u8)  [unwired: 1 out]
                            n228 = Bundle By Name(cluster=w608, "SyncEnable"=w604) -> (w609:T2)
                          }
                          frame "Sync Inverse" {
                            n229 = Match True/False String(2:"False", 3:"True", 4:w613) -> (0:w612:bool)  [unwired: 1 out]
                            n230 = Boolean To (0,1)(Boolean=w612) -> (0, 1=w611:i16)
                            n231 = To Unsigned Byte Integer(number=w611) -> (unsigned 8bit integer=w610:u8)
                            n232 = Bundle By Name(cluster=w616, "SyncInverse"=w610) -> (w617:T2)
                          }
                        }
                        n233 = local write "SOM_NewOutNSyncEnable"(w596) -> ()
                      }
                      frame "BurstLength 1".."BurstLength 9" {
                        n234 = Decimal String To Number(string=w619) -> (number=w618:i32)  [unwired: 2 in, 1 out]
                        n235 = Scan From String(format string="BurstLength %1d", input string=w620) -> (output 1=w624:i32)  [unwired: 3 in, 3 out]
                        n236 = Decrement(x=w624) -> (x-1=w623:i32)
                        n237 = local read "SOM_NewBurstLengthArray"() -> (w622:i32[])
                        n238 = Replace Array Subset(array=w622, new element=w618, index=w623) -> (w621:i32[])
                        n239 = local write "SOM_NewBurstLengthArray"(w621) -> ()
                      }
                      frame Default {
                      }
                    }
                  }
                  frame "SOMD" {
                    n240 = case shown="\"Divider\", \"MaskSync\", \"PreSync\"" w627 {
                      selector: w627 -> [_ w633 w651 w677 _]
                      tunnel: w626 -> [w629 w632 w650 w676 _]
                      frame "FreqTrigMode" {
                        n241 = Decimal String To Number(string=w629) -> (number=w628:i32)  [unwired: 2 in, 1 out]
                        n242 = local write "SOM_NewFreqTrigMode"(w628) -> ()
                      }
                      frame "Divider", "MaskSync", "PreSync" {
                        n243 = local read "SOMD_NewBurstValues"() -> (w630:T1)
                        n244 = case shown="\"MaskSync\"" w633 {
                          tunnel: w632 -> [_ w639 w644 w649]
                          tunnel: [w634 w638 w643 w648] -> w631
                          tunnel: w630 -> [w634 w637 w642 w647]
                          frame Default {
                          }
                          frame "Divider" {
                            n245 = Decimal String To Number(string=w639, default (0L)=u16 0 ("default (0 I32)")) -> (number=w636:u16)  [unwired: 1 in, 1 out]
                            n246 = Bundle By Name(cluster=w637, "Divider"=w636) -> (w638:T1)
                          }
                          frame "PreSync" {
                            n247 = Decimal String To Number(string=w644, default (0L)=u8 0 ("default (0 I32)")) -> (number=w641:u8)  [unwired: 1 in, 1 out]
                            n248 = Bundle By Name(cluster=w642, "PreSync"=w641) -> (w643:T1)
                          }
                          frame "MaskSync" {
                            n249 = Decimal String To Number(string=w649, default (0L)=u8 0 ("default (0 I32)")) -> (number=w646:u8)  [unwired: 1 in, 1 out]
                            n250 = Bundle By Name(cluster=w647, "SyncMask"=w646) -> (w648:T1)
                          }
                        }
                        n251 = local write "SOMD_NewBurstValues"(w631) -> ()
                      }
                      frame "Output Enable", "Sync Enable", "Sync Inverse" {
                        n252 = local read "SOM_NewOutNSyncEnable"() -> (w652:T2)
                        n253 = case shown="\"Sync Inverse\"" w651 {
                          tunnel: [w654 w660 w666 w674] -> w653
                          tunnel: w652 -> [w654 w659 w665 w673]
                          tunnel: w650 -> [_ w658 w664 w670]
                          frame Default {
                          }
                          frame "Output Enable" {
                            n254 = Hexadecimal String To Number(string=w658, offset=2, default (0uL)=u8 0 ("default (0 U32)")) -> (number=w655:u8)  [unwired: 1 out]
                            n255 = Bundle By Name(cluster=w659, "OutEnable"=w655) -> (w660:T2)
                          }
                          frame "Sync Enable" {
                            n256 = Hexadecimal String To Number(string=w664, offset=2, default (0uL)=u8 0 ("default (0 U32)")) -> (number=w661:u8)  [unwired: 1 out]
                            n257 = Bundle By Name(cluster=w665, "SyncEnable"=w661) -> (w666:T2)
                          }
                          frame "Sync Inverse" {
                            n258 = Match True/False String(2:"False", 3:"True", 4:w670) -> (0:w669:bool)  [unwired: 1 out]
                            n259 = Boolean To (0,1)(Boolean=w669) -> (0, 1=w668:i16)
                            n260 = To Unsigned Byte Integer(number=w668) -> (unsigned 8bit integer=w667:u8)
                            n261 = Bundle By Name(cluster=w673, "SyncInverse"=w667) -> (w674:T2)
                          }
                        }
                        n262 = local write "SOM_NewOutNSyncEnable"(w653) -> ()
                      }
                      frame "BurstLength 1".."BurstLength 9" {
                        n263 = Decimal String To Number(string=w676) -> (number=w675:i32)  [unwired: 2 in, 1 out]
                        n264 = Scan From String(format string="BurstLength %1d", input string=w677) -> (output 1=w681:i32)  [unwired: 3 in, 3 out]
                        n265 = Decrement(x=w681) -> (x-1=w680:i32)
                        n266 = local read "SOM_NewBurstLengthArray"() -> (w679:i32[])
                        n267 = Replace Array Subset(array=w679, new element=w675, index=w680) -> (w678:i32[])
                        n268 = local write "SOM_NewBurstLengthArray"(w678) -> ()
                      }
                      frame Default {
                      }
                    }
                  }
                  frame "SLM" {
                    n269 = case shown="\"FreqTrigIdx\"" w684 {
                      tunnel: w683 -> [_ w688 w693 w702]
                      frame Default {
                      }
                      frame "FreqTrigIdx" {
                        n270 = Decimal String To Number(string=w688) -> (number=w685:i32)  [unwired: 2 in, 1 out]
                        n271 = local read "SLM_NewPulseParameters"() -> (w686:cluster{"Freq":i32, "PulseMode":u8})
                        n272 = Bundle By Name(cluster=w686, "Freq"=w685) -> (w687:cluster{"Freq":i32, "PulseMode":u8})
                        n273 = local write "SLM_NewPulseParameters"(w687) -> ()
                      }
                      frame "Pulse Mode" {
                        n274 = Match True/False String(2:"False", 3:"True", 4:w693) -> (0:w692:bool)  [unwired: 1 out]
                        n275 = Boolean To (0,1)(Boolean=w692) -> (0, 1=w694:i16)
                        n276 = To Unsigned Byte Integer(number=w694) -> (unsigned 8bit integer=w689:u8)
                        n277 = local read "SLM_NewPulseParameters"() -> (w691:cluster{"Freq":i32, "PulseMode":u8})
                        n278 = Bundle By Name(cluster=w691, "PulseMode"=w689) -> (w690:cluster{"Freq":i32, "PulseMode":u8})
                        n279 = local write "SLM_NewPulseParameters"(w690) -> ()
                      }
                      frame "Intensity" {
                        n280 = Fract/Exp String To Number(string=w702, default (0 dbl)=sgl 0.0) -> (number=w699:sgl)  [unwired: 2 in, 1 out]
                        n281 = Multiply(x=u16 10 ("y"), y=w699) -> (x*y=w698:sgl)
                        n282 = To Unsigned Word Integer(number=w698) -> (unsigned 16bit integer=w697:u16)
                        n283 = local write "SLM_NewIntensity"(w697) -> ()
                      }
                    }
                  }
                  frame "VIR", "VUV" {
                    n284 = Equal?(x="VIR", y=w705) -> (x = y?=w703:bool)
                    n285 = case shown="\"FreqDivIdx\"" w707 {
                      tunnel: w706 -> [_ w710 w715 w720 w724 w733]
                      tunnel: w703 -> [_ w708 w713 w718 w729 w736]
                      frame Default {
                      }
                      frame "TrigSrcIdx" {
                        n286 = Decimal String To Number(string=w710) -> (number=w709:i32)  [unwired: 2 in, 1 out]
                        n287 = case shown="True" w708 {
                          tunnel: w709 -> [w711 w712]
                          frame False {
                            n288 = local write "VUV_NewTrigSrcIdx"(w711) -> ()
                          }
                          frame True {
                            n289 = local write "VIR_NewTrigSrcIdx"(w712) -> ()
                          }
                        }
                      }
                      frame "FreqDivIdx" {
                        n290 = Decimal String To Number(string=w715) -> (number=w714:i32)  [unwired: 2 in, 1 out]
                        n291 = case shown="True" w713 {
                          tunnel: w714 -> [w716 w717]
                          frame False {
                            n292 = local write "VUV_NewFreqDivIdx"(w716) -> ()
                          }
                          frame True {
                            n293 = local write "VIR_NewFreqDivIdx"(w717) -> ()
                          }
                        }
                      }
                      frame "TrigLevel" {
                        n294 = Decimal String To Number(string=w720) -> (number=w719:i32)  [unwired: 2 in, 1 out]
                        n295 = case shown="True" w718 {
                          tunnel: w719 -> [w721 w722]
                          frame False {
                            n296 = local write "VUV_NewTriggerLevel"(w721) -> ()
                          }
                          frame True {
                            n297 = local write "VIR_NewTriggerLevel"(w722) -> ()
                          }
                        }
                      }
                      frame "Intensity" {
                        n298 = Fract/Exp String To Number(string=w724, default (0 dbl)=sgl 0.0) -> (number=w726:sgl)  [unwired: 2 in, 1 out]
                        n299 = Multiply(x=u16 10 ("y"), y=w726) -> (x*y=w725:sgl)
                        n300 = To Long Integer(number=w725) -> (32bit integer=w723:i32)
                        n301 = case shown="True" w729 {
                          tunnel: w723 -> [w730 w731]
                          frame False {
                            n302 = local write "VUV_NewIntensity"(w730) -> ()
                          }
                          frame True {
                            n303 = local write "VIR_NewIntensity"(w731) -> ()
                          }
                        }
                      }
                      frame "FanRunning" {
                        n304 = Match True/False String(2:"False", 3:"True", 4:w733) -> (0:w732:bool)  [unwired: 1 out]
                        n305 = case shown="True" w736 {
                          tunnel: w732 -> [w737 w738]
                          frame False {
                            n306 = local write "VUV_NewFanRunning"(w737) -> ()
                          }
                          frame True {
                            n307 = local write "VIR_NewFanRunning"(w738) -> ()
                          }
                        }
                      }
                    }
                    n308 = local write "IsVIRModule"(w703) -> ()
                  }
                  frame "PRI" {
                    n309 = case shown="\"WavelengthIdx\"" w740 {
                      tunnel: w739 -> [_ w742 w744 w746]
                      frame Default {
                      }
                      frame "OperModeIdx" {
                        n310 = Decimal String To Number(string=w742) -> (number=w741:i32)  [unwired: 2 in, 1 out]
                        n311 = local write "PRI_NewOpModeIdx"(w741) -> ()
                      }
                      frame "WavelengthIdx" {
                        n312 = Decimal String To Number(string=w744) -> (number=w743:i32)  [unwired: 2 in, 1 out]
                        n313 = local write "PRI_NewWLIdx"(w743) -> ()
                      }
                      frame "Intensity" {
                        n314 = Fract/Exp String To Number(string=w746, default (0 dbl)=sgl 0.0) -> (number=w748:sgl)  [unwired: 2 in, 1 out]
                        n315 = Multiply(x=u16 10 ("y"), y=w748) -> (x*y=w747:sgl)
                        n316 = To Unsigned Word Integer(number=w747) -> (unsigned 16bit integer=w745:u16)
                        n317 = local write "PRI_NewIntensity"(w745) -> ()
                      }
                    }
                  }
                }
              }
            }
            n318 = Format Into String(format string="\\s\\s\\s%-4s\\s%-14s=\\s%s\\r\\n", error in=w386, w394, w391, w392) -> (resulting string=w397:string, error out=w385:errorcluster)  [unwired: 1 in]
            n319 = local read "cDisplay"() -> (w398:string)
            n320 = Concatenate Strings(w398, w397) -> (w396:string)
            n321 = local write "cDisplay"(w396) -> ()
          }
        }
        frame Error {
          # "save original data in file, modify it,\nthen write data to \"New\" fields"
          n322 = Not Equal?(x=w753, y=w757) -> (x != y?=w754:bool)
          n323 = case shown="True" w754 {
            tunnel: w753 -> [_ w1025]
            tunnel: [w773 w1025] -> w752
            tunnel: w756 -> [w779 _]
            tunnel: w755 -> [w774 _]
            tunnel: w751 -> [w758 _]
            frame True {
              # "write"
              n324 = local read "ModTypFound"() -> (w778:T8)
              n325 = local read "SlotNrsFound"() -> (w776:T6)
              n326 = local read "ModTypAbbr"() -> (w772:T4)
              n327 = local read "SerNrsFound"() -> (w765:T7)
              n328 = Cluster To Array(cluster=w778) -> (array=w766:bool[])
              n329 = Array Size(array=w766) -> (size(s)=w777:i32)
              n330 = Cluster To Array(cluster=w772) -> (array=w771:string[])
              n331 = Cluster To Array(cluster=w765) -> (array=w764:string[])
              n332 = Cluster To Array(cluster=w776) -> (array=w775:i32[])
              n333 = Open/Create/Replace File(file path (use dialog)=w779, error in=errorcluster {"status"=FALSE, "code"=0, "source"=""} ("error in 2 (no error)"), operation (0:open)=T10."create", access (0:read/write)=enum16{"read/write", "read-only", "write-only"}."write-only") -> (refnum out=w770:refnum<file>, error out=w769:errorcluster)  [unwired: 2 in, 1 out]
              n334 = for {
                N: w777 -> [_]
                tunnel: w766 -> [w783] mode=indexing
                tunnel: w775 -> [w794] mode=indexing
                tunnel: w774 -> [w793]
                tunnel: w771 -> [w790] mode=indexing
                tunnel: w769 -> [w792]
                tunnel: [w791] -> w768
                shift-right: [w789] -> w760
                shift-left: "" -> [w784]
                tunnel: w758 -> [w788] mode=indexing
                tunnel: w764 -> [w787] mode=indexing
                i -> [w786]
                n335 = case shown="True" w783 {
                  tunnel: w794 -> [_ w805]
                  tunnel: w793 -> [_ w804]
                  tunnel: w790 -> [_ w803]
                  tunnel: w792 -> [w799 w806]
                  tunnel: [w799 w801] -> w791
                  tunnel: w788 -> [w796 _]
                  tunnel: w787 -> [_ w802]
                  tunnel: w786 -> [_ w807]
                  tunnel: [w795 w800] -> w785
                  frame False {
                    n336 = Format Into String(format string="%1$4s ModuleFound   =        False\\r\\n", initial string="", w796) -> (resulting string=w795:string)  [unwired: 1 in, 1 out]
                  }
                  frame True {
                    n337 = case shown="0" w807 {
                      selector: w807 -> [_ _ _ w977 _]
                      tunnel: w806 -> [w809 w815 w937 w979 w1013]
                      tunnel: [w809 w821 w943 w984 w1014] -> w801
                      tunnel: ["" w818 w942 w983 w1011] -> w800
                      tunnel: w805 -> [_ w812 w934 w955 w1016]
                      tunnel: w804 -> [_ w813 w935 w954 w1019]
                      tunnel: w803 -> [_ w811 w941 w982 w1017]
                      tunnel: w802 -> [_ w820 w940 w981 w1015]
                      frame -1, Default {
                      }
                      frame 0 {
                        n338 = local read "IsSOMDModule"() -> (w817:bool)
                        n339 = case shown="True" w817 {
                          tunnel: [w850 w895] -> w816
                          tunnel: w815 -> [w858 w903]
                          tunnel: [w849 w894] -> w814
                          tunnel: w813 -> [w854 w899]
                          tunnel: w812 -> [w852 w897]
                          tunnel: w811 -> [w832 w877]
                          frame False {
                            w829 = 2
                            w830 = 1
                            w851 = "%1$4s FreqTrigMode  =        %2$1d\\r\\n%1$4s Divider       =      %3$3d\\r\\n%1$4s PreSync       =      %4$3d\\r\\n%1$4s MaskSync      =      %5$3d\\r\\n%1$4s Output Enable =     0x%6$02X\\r\\n%1$4s Sync Enable   =     0x%7$02X\\r\\n%1$4s Sync Inverse  =        %8$s\\r\\n%s"  # %1$4s FreqTrigMode  =        %2$1d\r\n%1$4s Divider       =      %3$3d\r\n%1$4s PreSync       =      %4$3d\r\n%1$4s MaskSync      =      %5$3d\r\n%1$4s Output Enable =     0x%6$02X\r\n%1$4s Sync Enable   =     0x%7$02X\r\n%1$4s Sync Inverse  =        %8$s\r\n%s
                            n340 = call "SOM Get Freq Trig Mode.vi"("error in (no error)"=w858, "SlotId"=w852, "DevIdx"=w854) -> ("error out"=w857:errorcluster, "FreqTrigMode"=w848:i32)  [unwired: 1 out]
                            n341 = call "SOM Get Burst Values.vi"("error in (no error)"=w857, "SlotId"=w852, "DevIdx"=w854) -> ("error out"=w856:errorcluster, "SOM Burst Values"=w847:T3)  [unwired: 1 out]
                            n342 = Unbundle By Name(w847) -> ("Divider"=w846:u8, "PreSync"=w845:u8, "SyncMask"=w844:u8)
                            n343 = call "SOM Get Out N Sync Enable.vi"("error in (no error)"=w856, "SlotId"=w852, "DevIdx"=w854) -> ("error out"=w855:errorcluster, "SOM Out N Sync Enable"=w843:T2)  [unwired: 1 out]
                            n344 = Unbundle By Name(w843) -> ("OutEnable"=w842:u8, "SyncEnable"=w841:u8, "SyncInverse"=w840:enum8{"Standard_Sync_Mask", "Inverse_Sync_Mask"})
                            n345 = Not Equal To 0?(x=w840) -> (x != 0?=w839:bool)
                            n346 = call "SOM Get Burst Length Array.vi"("error in (no error)"=w855, "SlotId"=w852, "DevIdx"=w854) -> ("error out"=w826:errorcluster, "SOM Burst Length Array"=w831:i32[])  [unwired: 1 out]
                            n347 = for {
                              N: 8 -> [_]
                              tunnel: w831 -> [w860] mode=indexing
                              shift-right: [w865] -> w833
                              shift-left: "" -> [w863]
                              tunnel: w832 -> [w862]
                              i -> [w861]
                              n348 = Increment(x=w861) -> (x+1=w859:i32)
                              n349 = Format Into String(format string="%4s BurstLength %d = %8d\\r\\n", initial string=w863, w862, w859, w860) -> (resulting string=w865:string)  [unwired: 1 in, 1 out]
                            }
                            n350 = Index Array(array=w831, index #1=w830, index #2=w829) -> (element #1=w827:i32, element #2=w828:i32)
                            n351 = Select(t="True", s=w839, f="False") -> (s? t:f=w838:string)
                            n352 = Format Into String(format string=w851, initial string="", error in=w826, w832, w848, w846, w845, w844, w842, w841, w838, w833) -> (resulting string=w850:string, error out=w849:errorcluster)
                            n353 = Replace Array Subset(array=w831, new element #1=w828, index #1=w830, new element #2=w827, index #2=w829) -> (w825:i32[])
                            n354 = local write "SOM_NewBurstLengthArray"(w825) -> ()
                            n355 = local write "SOM_NewOutNSyncEnable"(T2 {"OutEnable"=165, "SyncEnable"=147, "SyncInverse"=enum."Inverse_Sync_Mask"} ("SOM_NewOutNSyncEnable")) -> ()
                            n356 = local write "SOM_NewFreqTrigMode"(4 ("SOM_NewFreqTrigMode")) -> ()
                            n357 = local write "SOM_NewBurstValues"(T3 {"Divider"=200, "PreSync"=10, "SyncMask"=1} ("SOM_NewBurstValues")) -> ()
                          }
                          frame True {
                            w875 = 2
                            w876 = 1
                            w896 = "%1$4s FreqTrigMode  =        %2$1d\\r\\n%1$4s Divider       =      %3$3d\\r\\n%1$4s PreSync       =      %4$3d\\r\\n%1$4s MaskSync      =      %5$3d\\r\\n%1$4s Output Enable =     0x%6$02X\\r\\n%1$4s Sync Enable   =     0x%7$02X\\r\\n%1$4s Sync Inverse  =        %8$s\\r\\n%s"  # %1$4s FreqTrigMode  =        %2$1d\r\n%1$4s Divider       =      %3$3d\r\n%1$4s PreSync       =      %4$3d\r\n%1$4s MaskSync      =      %5$3d\r\n%1$4s Output Enable =     0x%6$02X\r\n%1$4s Sync Enable   =     0x%7$02X\r\n%1$4s Sync Inverse  =        %8$s\r\n%s
                            n358 = call "SOMD Get Freq Trig Mode.vi"("DevIdx"=w899, "SlotId"=w897, "error in (no error)"=w903) -> ("FreqTrigMode"=w893:i32, "Synchronize"=w867:bool, "error out"=w902:errorcluster)  [unwired: 1 out]
                            n359 = call "SOMD Get Burst Values.vi"("error in (no error)"=w902, "SlotId"=w897, "DevIdx"=w899) -> ("error out"=w901:errorcluster, "SOMD Burst Values"=w892:T1)  [unwired: 1 out]
                            n360 = Unbundle By Name(w892) -> ("Divider"=w891:u16, "PreSync"=w890:u8, "SyncMask"=w889:u8)
                            n361 = call "SOMD Get Out N Sync Enable.vi"("error in (no error)"=w901, "SlotId"=w897, "DevIdx"=w899) -> ("error out"=w900:errorcluster, "SOMD Out N Sync Enable"=w888:T2)  [unwired: 1 out]
                            n362 = Unbundle By Name(w888) -> ("OutEnable"=w887:u8, "SyncEnable"=w886:u8, "SyncInverse"=w885:enum8{"Standard_Sync_Mask", "Inverse_Sync_Mask"})
                            n363 = Not Equal To 0?(x=w885) -> (x != 0?=w884:bool)
                            n364 = call "SOMD Get Burst Length Array.vi"("error in (no error)"=w900, "SlotId"=w897, "DevIdx"=w899) -> ("error out"=w872:errorcluster, "SOMD Burst Length Array"=w866:i32[])  [unwired: 1 out]
                            n365 = for {
                              N: 8 -> [_]
                              tunnel: w866 -> [w905] mode=indexing
                              shift-right: [w910] -> w878
                              shift-left: "" -> [w908]
                              tunnel: w877 -> [w907]
                              i -> [w906]
                              n366 = Increment(x=w906) -> (x+1=w904:i32)
                              n367 = Format Into String(format string="%4s BurstLength %d = %8d\\r\\n", initial string=w908, w907, w904, w905) -> (resulting string=w910:string)  [unwired: 1 in, 1 out]
                            }
                            n368 = Index Array(array=w866, index #1=w876, index #2=w875) -> (element #1=w873:i32, element #2=w874:i32)
                            n369 = Select(t="True", s=w884, f="False") -> (s? t:f=w883:string)
                            n370 = Format Into String(format string=w896, initial string="", error in=w872, w877, w893, w891, w890, w889, w887, w886, w883, w878) -> (resulting string=w895:string, error out=w894:errorcluster)
                            n371 = Replace Array Subset(array=w866, new element #1=w874, index #1=w876, new element #2=w873, index #2=w875) -> (w871:i32[])
                            n372 = local write "SOM_NewBurstLengthArray"(w871) -> ()
                            n373 = local write "SOM_NewOutNSyncEnable"(T2 {"OutEnable"=165, "SyncEnable"=147, "SyncInverse"=enum."Inverse_Sync_Mask"} ("SOM_NewOutNSyncEnable")) -> ()
                            n374 = local write "SOM_NewFreqTrigMode"(4 ("SOM_NewFreqTrigMode")) -> ()
                            n375 = local write "SOMD_NewBurstValues"(T1 {"Divider"=300, "PreSync"=10, "SyncMask"=1} ("SOMD_NewBurstValues")) -> ()
                            n376 = local write "SOMD_Sync"(w867) -> ()
                          }
                        }
                        n377 = Format Into String(format string="%1$4s ModuleFound   =        True\\r\\n%1$4s SlotID        =      %2$03d\\r\\n%1$4s SerialNumber  = %3$8s\\r\\n%s", initial string="", error in=w814, w811, w812, w820, w816) -> (resulting string=w818:string, error out=w821:errorcluster)
                      }
                      frame 1 {
                        n378 = call "SLM Get Intensity Fine Step.vi"("error in (no error)"=w937, "SlotId"=w934, "DevIdx"=w935) -> ("error out"=w936:errorcluster, "Intensity"=w918:u16)  [unwired: 1 out]
                        n379 = call "SLM Get Pulse Parameters.vi"("error in (no error)"=w936, "SlotId"=w934, "DevIdx"=w935) -> ("error out"=w933:errorcluster, "SLM Pulse Parameters"=w915:T13)  [unwired: 1 out]
                        n380 = Unbundle By Name(w915) -> ("Freq"=w923:i32, "PulseMode"=w932:u8)
                        n381 = Divide(x=w918, y=u16 10 ("Intensity")) -> (x/y=w927:dbl)
                        n382 = Not Equal To 0?(x=w932) -> (x != 0?=w921:bool)
                        n383 = Select(t="True" ("input 5"), s=w921, f="False") -> (s? t:f=w929:string)
                        n384 = Not(x=w921) -> (.not. x?=w922:bool)
                        n385 = Boolean To (0,1)(Boolean=w922) -> (0, 1=w916:i16)
                        n386 = To Unsigned Word Integer(number=1000) -> (unsigned 16bit integer=w919:u16)
                        n387 = Add(x=2, y=w923) -> (x+y=w925:i32)
                        n388 = To Unsigned Byte Integer(number=w916) -> (unsigned 8bit integer=w912:u8)
                        n389 = Quotient & Remainder(x=w925, y=8) -> (x-y*floor(x/y)=w911:i32)  [unwired: 1 out]
                        n390 = Subtract(x=w919, y=w918) -> (x-y=w917:u16)
                        n391 = Format Into String(format string="%1$4s ModuleFound   =        True\\r\\n%1$4s SlotID        =      %2$03d\\r\\n%1$4s SerialNumber  = %3$8s\\r\\n%1$4s FreqTrigIdx   =        %4$1d\\r\\n%1$4s Pulse Mode    =        %5$s\\r\\n%1$4s Intensity     =      %6$5.1f %%\\r\\n", initial string="", error in=w933, w941, w934, w940, w923, w929, w927) -> (resulting string=w942:string, error out=w943:errorcluster)
                        n392 = local read "SLM_NewPulseParameters"() -> (w913:cluster{"Freq":i32, "PulseMode":u8})
                        n393 = Bundle By Name(cluster=w913, "Freq"=w911, "PulseMode"=w912) -> (w914:cluster{"Freq":i32, "PulseMode":u8})
                        n394 = local write "SLM_NewPulseParameters"(w914) -> ()
                        n395 = local write "SLM_NewIntensity"(w917) -> ()
                      }
                      frame 2, 3 {
                        w959 = 2
                        w963 = 1
                        n396 = call "VUV_VIR Get Trigger Data.vi"("DevIdx"=w954, "SlotId"=w955, "error in (no error)"=w979) -> ("MainTrigSrcIdx"=w950:i32, "MainFreqDivIdx"=w956:i32, "error out"=w973:errorcluster, "TrigLevel"=w968:i32)  [unwired: 1 out]
                        n397 = call "VUV_VIR Get Tigger Level Range.vi"("DevIdx"=w954, "SlotId"=w955, "error in (no error)"=w973) -> ("UpperTL"=w971:i32, "LowerTL"=w970:i32, "error out"=w972:errorcluster)  [unwired: 2 out]
                        n398 = call "VUV_VIR Get Intensity.vi"("error in (no error)"=w972, "SlotId"=w955, "DevIdx"=w954) -> ("error out"=w976:errorcluster, "Intensity"=w951:i32)  [unwired: 1 out]
                        n399 = call "VUV_VIR Get Fan.vi"("error in (no error)"=w976, "SlotId"=w955, "DevIdx"=w954) -> ("error out"=w944:errorcluster, "FanRunning"=w946:bool)  [unwired: 1 out]
                        n400 = Select(t="True" ("input 5"), s=w946, f="False") -> (s? t:f=w945:string)
                        n401 = Divide(x=w951, y=u16 10 ("Intensity")) -> (x/y=w974:dbl)
                        n402 = Equal?(x=3 ("y"), y=w977) -> (x = y?=w966:bool)
                        n403 = Equal?(x=w950, y=w963) -> (x = y?=w964:bool)
                        n404 = Equal?(x=w956, y=w959) -> (x = y?=w960:bool)
                        n405 = Not(x=w946) -> (.not. x?=w949:bool)
                        n406 = Subtract(x=50, y=w968) -> (x-y=w967:i32)
                        n407 = Subtract(x=1000, y=w951) -> (x-y=w952:i32)
                        n408 = Select(t=1, s=w960, f=w959) -> (s? t:f=w957:i32)
                        n409 = Select(t=0, s=w964, f=w963) -> (s? t:f=w961:i32)
                        n410 = In Range and Coerce(upper limit=w971, x=w967, lower limit=w970) -> (coerced(x)=w965:i32)  [unwired: 1 out]
                        n411 = case shown="False" w966 {
                          tunnel: w965 -> [w986 w995]
                          tunnel: w961 -> [w987 w994]
                          tunnel: w957 -> [w988 w993]
                          tunnel: w952 -> [w989 w992]
                          tunnel: w949 -> [w990 w991]
                          frame False {
                            n412 = local write "VUV_NewTriggerLevel"(w986) -> ()
                            n413 = local write "VUV_NewFanRunning"(w990) -> ()
                            n414 = local write "VUV_NewFreqDivIdx"(w988) -> ()
                            n415 = local write "VUV_NewTrigSrcIdx"(w987) -> ()
                            n416 = local write "VUV_NewIntensity"(w989) -> ()
                          }
                          frame True {
                            n417 = local write "VIR_NewTriggerLevel"(w995) -> ()
                            n418 = local write "VIR_NewFanRunning"(w991) -> ()
                            n419 = local write "VIR_NewFreqDivIdx"(w993) -> ()
                            n420 = local write "VIR_NewTrigSrcIdx"(w994) -> ()
                            n421 = local write "VIR_NewIntensity"(w992) -> ()
                          }
                        }
                        n422 = Format Into String(format string="%1$4s ModuleFound   =        True\\r\\n%1$4s SlotID        =      %2$03d\\r\\n%1$4s SerialNumber  = %3$8s\\r\\n%1$4s TrigSrcIdx    =      %4$3d\\r\\n%1$4s FreqDivIdx    =      %5$3d\\r\\n%1$4s TrigLevel     =    %6$5d\\r\\n%1$4s Intensity     =      %7$5.1f %%\\r\\n%1$4s FanRunning    =        %8$s\\r\\n", initial string="", error in=w944, w982, w955, w981, w950, w956, w968, w974, w945) -> (resulting string=w983:string, error out=w984:errorcluster)
                        n423 = local write "IsVIRModule"(w966) -> ()
                      }
                      frame 4 {
                        n424 = local read "PRIConst"() -> (w1010:T5)
                        n425 = Unbundle By Name(w1010) -> ("PrimaOpModBroad"=w1000:i32, "PrimaOpModNarrow"=w1008:i32, "PrimaWLCount"=w1004:i32)
                        n426 = call "PRI Get Operation Mode.vi"("error in (no error)"=w1013, "SlotId"=w1016, "DevIdx"=w1019) -> ("error out"=w1021:errorcluster, "OpMode_Idx"=w1007:i32)  [unwired: 1 out]
                        n427 = call "PRI Get Wavelength Index.vi"("error in (no error)"=w1021, "SlotId"=w1016, "DevIdx"=w1019) -> ("error out"=w1022:errorcluster, "Wavelength_Idx"=w1006:i32)  [unwired: 1 out]
                        n428 = call "PRI Get Intensity.vi"("error in (no error)"=w1022, "Wavelength Idx"=w1006, "SlotId"=w1016, "DevIdx"=w1019) -> ("error out"=w1023:errorcluster, "Intensity"=w1003:u16)  [unwired: 1 out]
                        n429 = Divide(x=w1003, y=u16 10 ("Intensity")) -> (x/y=w999:dbl)
                        n430 = To Unsigned Word Integer(number=1000) -> (unsigned 16bit integer=w1001:u16)
                        n431 = Not Equal?(x=w1000, y=w1007) -> (x != y?=w1009:bool)
                        n432 = Increment(x=w1006) -> (x+1=w1005:i32)
                        n433 = Select(t=w1000, s=w1009, f=w1008) -> (s? t:f=w998:i32)
                        n434 = Subtract(x=w1001, y=w1003) -> (x-y=w996:u16)
                        n435 = Quotient & Remainder(x=w1005, y=w1004) -> (x-y*floor(x/y)=w997:i32)  [unwired: 1 out]
                        n436 = Format Into String(format string="%1$4s ModuleFound   =        True\\r\\n%1$4s SlotID        =      %2$03d\\r\\n%1$4s SerialNumber  = %3$8s\\r\\n%1$4s OperModeIdx   =        %4$1d\\r\\n%1$4s WavelengthIdx =        %5$1d\\r\\n%1$4s Intensity     =      %6$5.1f %%\\r\\n", initial string="", error in=w1023, w1017, w1016, w1015, w1007, w1006, w999) -> (resulting string=w1011:string, error out=w1014:errorcluster)
                        n437 = local write "PRI_NewOpModeIdx"(w998) -> ()
                        n438 = local write "PRI_NewIntensity"(w996) -> ()
                        n439 = local write "PRI_NewWLIdx"(w997) -> ()
                      }
                    }
                  }
                }
                n440 = Concatenate Strings(w784, w785) -> (w789:string)
              }
              n441 = local read "cDisplay"() -> (w763:string)
              n442 = Concatenate Strings(w763, "original data as stored in file 'OrigData.txt': \n", "\r\n", w760) -> (w762:string)
              n443 = local write "cDisplay"(w762) -> ()
              n444 = Write to Text File(file (use dialog)=w770, text=w760, error in=w768) -> (error out=w773:errorcluster)  [unwired: 1 in, 2 out]
            }
            frame False {
              # "Error"
              n445 = local write "cDisplay"("\n     You probably tried to start this demo in a write protected directory.\n     Demo execution aborted.\n") -> ()
            }
          }
        }
      }
    }
    frame #5 {
      w1029 = "\r\n"
      n446 = local read "SlotNrsFound"() -> (w1038:T6)
      n447 = local read "ModTypAbbr"() -> (w1040:T4)
      n448 = local read "ModTypFound"() -> (w1036:T8)
      n449 = Cluster To Array(cluster=w1036) -> (array=w1037:bool[])
      n450 = Cluster To Array(cluster=w1040) -> (array=w1041:string[])
      n451 = Cluster To Array(cluster=w1038) -> (array=w1039:i32[])
      n452 = Array Size(array=w1037) -> (size(s)=w1035:i32)
      n453 = for {
        N: w1035 -> [_]
        tunnel: w1037 -> [w1053] mode=indexing
        tunnel: w1031 -> [w1051]
        tunnel: w1039 -> [w1052] mode=indexing
        shift-right: [w1048] -> w1032
        shift-left: w1033 -> [w1049]
        shift-right: [w1046] -> w1028
        shift-left: "" -> [w1047]
        tunnel: w1041 -> [w1045] mode=indexing
        i -> [w1050]
        n454 = case shown="True" w1053 {
          tunnel: w1052 -> [_ w1060]
          tunnel: w1051 -> [_ w1061]
          tunnel: w1050 -> [_ w1062]
          tunnel: w1049 -> [w1055 w1059]
          tunnel: [w1055 w1058] -> w1048
          tunnel: w1045 -> [_ w1057]
          tunnel: ["" w1056] -> w1044
          frame False {
          }
          frame True {
            n455 = case shown="0" w1062 {
              selector: w1062 -> [_ _ _ w1174 _]
              tunnel: w1061 -> [_ w1070 w1149 w1172 w1201]
              tunnel: w1060 -> [_ w1067 w1148 w1171 w1200]
              tunnel: w1059 -> [w1064 w1069 w1151 w1170 w1199]
              tunnel: [w1064 w1068 w1147 w1163 w1186] -> w1058
              tunnel: w1057 -> [_ w1065 w1142 w1162 w1188]
              tunnel: ["" w1066 w1143 w1165 w1195] -> w1056
              frame -1, Default {
              }
              frame 0 {
                n456 = local read "IsSOMDModule"() -> (w1071:bool)
                n457 = case shown="False" w1071 {
                  tunnel: w1070 -> [w1097 w1128]
                  tunnel: w1067 -> [w1096 w1127]
                  tunnel: w1069 -> [w1102 w1132]
                  tunnel: [w1072 w1119] -> w1068
                  tunnel: [w1093 w1118] -> w1066
                  tunnel: w1065 -> [w1092 w1121]
                  frame True {
                    w1094 = "%1$4s FreqTrigMode  =>        %2$1d\\r\\n%1$4s Divider       =>    %3$5d\\r\\n%1$4s PreSync       =>      %4$3d\\r\\n%1$4s MaskSync      =>      %5$3d\\r\\n%1$4s Output Enable =>     0x%6$02X\\r\\n%1$4s Sync Enable   =>     0x%7$02X\\r\\n%1$4s Sync Inverse  =>        %8$s\\r\\n%1$4s BurstLength 1 => %9$8d\\r\\n%1$4s BurstLength 2 => %10$8d\\r\\n"  # %1$4s FreqTrigMode  =>        %2$1d\r\n%1$4s Divider       =>    %3$5d\r\n%1$4s PreSync       =>      %4$3d\r\n%1$4s MaskSync      =>      %5$3d\r\n%1$4s Output Enable =>     0x%6$02X\r\n%1$4s Sync Enable   =>     0x%7$02X\r\n%1$4s Sync Inverse  =>        %8$s\r\n%1$4s BurstLength 1 => %9$8d\r\n%1$4s BurstLength 2 => %10$8d\r\n
                    n458 = local read "SOM_NewBurstLengthArray"() -> (w1076:i32[])
                    n459 = local read "SOM_NewOutNSyncEnable"() -> (w1086:T2)
                    n460 = local read "SOM_NewFreqTrigMode"() -> (w1091:i32)
                    n461 = local read "SOMD_NewBurstValues"() -> (w1090:T1)
                    n462 = local read "SOMD_Sync"() -> (w1101:bool)
                    n463 = Unbundle(w1086) -> ("OutEnable"=w1085:u8, "SyncEnable"=w1084:u8, "SyncInverse"=w1083:enum8{"Standard_Sync_Mask", "Inverse_Sync_Mask"})
                    n464 = Index Array(array=w1076, index #1=1, index #2=2) -> (element #1=w1075:i32, element #2=w1074:i32)
                    n465 = Not Equal To 0?(x=w1083) -> (x != 0?=w1082:bool)
                    n466 = call "SOMD Set Freq Trig Mode.vi"("DevIdx"=w1097, "SlotId"=w1096, "FreqTrigMode"=w1091, "error in (no error)"=w1102, "Synchronize"=w1101) -> ("error out"=w1100:errorcluster)  [unwired: 1 out]
                    n467 = call "SOMD Set Burst Values.vi"("error in (no error)"=w1100, "SOMD Burst Values"=w1090, "SlotId"=w1096, "DevIdx"=w1097) -> ("error out"=w1099:errorcluster)  [unwired: 1 out]
                    n468 = call "SOMD Set Out N Sync Enable.vi"("error in (no error)"=w1099, "SOM Out N Sync Enable"=w1086, "SlotId"=w1096, "DevIdx"=w1097) -> ("error out"=w1098:errorcluster)  [unwired: 1 out]
                    n469 = call "SOMD Set Burst Length Array.vi"("error in (no error)"=w1098, "SOMD Burst Length Array"=w1076, "SlotId"=w1096, "DevIdx"=w1097) -> ("error out"=w1073:errorcluster)  [unwired: 1 out]
                    n470 = Unbundle(w1090) -> ("Divider"=w1089:u16, "PreSync"=w1088:u8, "SyncMask"=w1087:u8)
                    n471 = Select(t="True", s=w1082, f="False") -> (s? t:f=w1079:string)
                    n472 = Format Into String(format string=w1094, initial string="", error in=w1073, w1092, w1091, w1089, w1088, w1087, w1085, w1084, w1079, w1075, w1074) -> (resulting string=w1093:string, error out=w1072:errorcluster)
                  }
                  frame False {
                    w1125 = "%1$4s FreqTrigMode  =>        %2$1d\\r\\n%1$4s Divider       =>      %3$3d\\r\\n%1$4s PreSync       =>      %4$3d\\r\\n%1$4s MaskSync      =>      %5$3d\\r\\n%1$4s Output Enable =>     0x%6$02X\\r\\n%1$4s Sync Enable   =>     0x%7$02X\\r\\n%1$4s Sync Inverse  =>        %8$s\\r\\n%1$4s BurstLength 1 => %9$8d\\r\\n%1$4s BurstLength 2 => %10$8d\\r\\n"  # %1$4s FreqTrigMode  =>        %2$1d\r\n%1$4s Divider       =>      %3$3d\r\n%1$4s PreSync       =>      %4$3d\r\n%1$4s MaskSync      =>      %5$3d\r\n%1$4s Output Enable =>     0x%6$02X\r\n%1$4s Sync Enable   =>     0x%7$02X\r\n%1$4s Sync Inverse  =>        %8$s\r\n%1$4s BurstLength 1 => %9$8d\r\n%1$4s BurstLength 2 => %10$8d\r\n
                    n473 = local read "SOM_NewBurstLengthArray"() -> (w1106:i32[])
                    n474 = local read "SOM_NewOutNSyncEnable"() -> (w1112:T2)
                    n475 = local read "SOM_NewFreqTrigMode"() -> (w1117:i32)
                    n476 = local read "SOM_NewBurstValues"() -> (w1116:T3)
                    n477 = Unbundle(w1112) -> ("OutEnable"=w1111:u8, "SyncEnable"=w1110:u8, "SyncInverse"=w1115:enum8{"Standard_Sync_Mask", "Inverse_Sync_Mask"})
                    n478 = Index Array(array=w1106, index #1=1, index #2=2) -> (element #1=w1105:i32, element #2=w1104:i32)
                    n479 = Not Equal To 0?(x=w1115) -> (x != 0?=w1114:bool)
                    n480 = call "SOM Set Freq Trig Mode.vi"("error in (no error)"=w1132, "FreqTrigMode"=w1117, "SlotId"=w1127, "DevIdx"=w1128) -> ("error out"=w1131:errorcluster)  [unwired: 1 out]
                    n481 = call "SOM Set Burst Values.vi"("error in (no error)"=w1131, "SOM Burst Values"=w1116, "SlotId"=w1127, "DevIdx"=w1128) -> ("error out"=w1130:errorcluster)  [unwired: 1 out]
                    n482 = call "SOM Set Out N Sync Enable.vi"("error in (no error)"=w1130, "SOM Out N Sync Enable"=w1112, "SlotId"=w1127, "DevIdx"=w1128) -> ("error out"=w1129:errorcluster)  [unwired: 1 out]
                    n483 = call "SOM Set Burst Length Array.vi"("error in (no error)"=w1129, "SOM Burst Length Array"=w1106, "SlotId"=w1127, "DevIdx"=w1128) -> ("error out"=w1120:errorcluster)  [unwired: 1 out]
                    n484 = Unbundle(w1116) -> ("Divider"=w1124:u8, "PreSync"=w1123:u8, "SyncMask"=w1122:u8)
                    n485 = Select(t="True", s=w1114, f="False") -> (s? t:f=w1109:string)
                    n486 = Format Into String(format string=w1125, initial string="", error in=w1120, w1121, w1117, w1124, w1123, w1122, w1111, w1110, w1109, w1105, w1104) -> (resulting string=w1118:string, error out=w1119:errorcluster)
                  }
                }
              }
              frame 1 {
                n487 = local read "SLM_NewPulseParameters"() -> (w1146:cluster{"Freq":i32, "PulseMode":u8})
                n488 = local read "SLM_NewIntensity"() -> (w1134:u16)
                n489 = Unbundle By Name(w1146) -> ("Freq"=w1141:i32, "PulseMode"=w1136:u8)
                n490 = Divide(x=w1134, y=u16 10 ("Intensity")) -> (x/y=w1133:dbl)
                n491 = call "SLM Set Intensity Fine Step.vi"("error in (no error)"=w1151, "Intensity"=w1134, "SlotId"=w1148, "DevIdx"=w1149) -> ("error out"=w1150:errorcluster)  [unwired: 1 out]
                n492 = call "SLM Set Pulse Parameters.vi"("error in (no error)"=w1150, "SLM Pulse Parameters"=w1146, "SlotId"=w1148, "DevIdx"=w1149) -> ("error out"=w1147:errorcluster)  [unwired: 1 out]
                n493 = Not Equal To 0?(x=w1136) -> (x != 0?=w1138:bool)
                n494 = Select(t="True" ("input 5"), s=w1138, f="False") -> (s? t:f=w1135:string)
                n495 = Format Into String(format string="%1$4s FreqTrigIdx   =>        %2$1d\\r\\n%1$4s Pulse Mode    =>        %3$s\\r\\n%1$4s Intensity     =>      %4$5.1f %%\\r\\n", initial string="", w1142, w1141, w1135, w1133) -> (resulting string=w1143:string)  [unwired: 1 in, 1 out]
              }
              frame 2, 3 {
                n496 = Equal?(x=3 ("y"), y=w1174) -> (x = y?=w1173:bool)
                n497 = case shown="True" w1173 {
                  tunnel: [w1180 w1185] -> w1153
                  tunnel: [w1179 w1184] -> w1154
                  tunnel: [w1178 w1183] -> w1152
                  tunnel: [w1177 w1182] -> w1158
                  tunnel: [w1176 w1181] -> w1156
                  frame False {
                    n498 = local read "VUV_NewTriggerLevel"() -> (w1178:i32)
                    n499 = local read "VUV_NewFanRunning"() -> (w1176:bool)
                    n500 = local read "VUV_NewFreqDivIdx"() -> (w1180:i32)
                    n501 = local read "VUV_NewTrigSrcIdx"() -> (w1179:i32)
                    n502 = local read "VUV_NewIntensity"() -> (w1177:i32)
                  }
                  frame True {
                    n503 = local read "VIR_NewTriggerLevel"() -> (w1183:i32)
                    n504 = local read "VIR_NewFanRunning"() -> (w1181:bool)
                    n505 = local read "VIR_NewFreqDivIdx"() -> (w1185:i32)
                    n506 = local read "VIR_NewTrigSrcIdx"() -> (w1184:i32)
                    n507 = local read "VIR_NewIntensity"() -> (w1182:i32)
                  }
                }
                n508 = Divide(x=w1158, y=u16 10 ("Intensity")) -> (x/y=w1157:dbl)
                n509 = Select(t="True" ("input 5"), s=w1156, f="False") -> (s? t:f=w1155:string)
                n510 = call "VUV_VIR Set Trigger Data.vi"("TrigLevel"=w1152, "MainFreqDivIdx"=w1153, "error in (no error)"=w1170, "MainTrigSrcIdx"=w1154, "SlotId"=w1171, "DevIdx"=w1172) -> ("error out"=w1169:errorcluster)  [unwired: 1 out]
                n511 = call "VUV_VIR Set Intensity.vi"("error in (no error)"=w1169, "Intensity"=w1158, "SlotId"=w1171, "DevIdx"=w1172) -> ("error out"=w1168:errorcluster)  [unwired: 1 out]
                n512 = call "VUV_VIR Set Fan.vi"("error in (no error)"=w1168, "FanRunning"=w1156, "SlotId"=w1171, "DevIdx"=w1172) -> ("error out"=w1164:errorcluster)  [unwired: 1 out]
                n513 = Format Into String(format string="%1$4s TrigSrcIdx    =>      %2$3d\\r\\n%1$4s FreqDivIdx    =>      %3$3d\\r\\n%1$4s TrigLevel     =>    %4$5d\\r\\n%1$4s Intensity     =>      %5$5.1f %%\\r\\n%1$4s FanRunning    =>        %6$s\\r\\n", initial string="", error in=w1164, w1162, w1154, w1153, w1152, w1157, w1155) -> (resulting string=w1165:string, error out=w1163:errorcluster)
              }
              frame 4 {
                n514 = local read "PRI_NewOpModeIdx"() -> (w1189:i32)
                n515 = local read "PRI_NewIntensity"() -> (w1192:u16)
                n516 = local read "PRI_NewWLIdx"() -> (w1190:i32)
                n517 = Divide(x=w1192, y=u16 10 ("Intensity")) -> (x/y=w1191:dbl)
                n518 = call "PRI Set Operation Mode.vi"("error in (no error)"=w1199, "OpMode_Idx"=w1189, "SlotId"=w1200, "DevIdx"=w1201) -> ("error out"=w1198:errorcluster)  [unwired: 1 in, 1 out]
                n519 = call "PRI Set Wavelength Index.vi"("error in (no error)"=w1198, "Wavelength_Idx"=w1190, "SlotId"=w1200, "DevIdx"=w1201) -> ("error out"=w1197:errorcluster)  [unwired: 1 in, 1 out]
                n520 = call "PRI Set Intensity.vi"("DevIdx"=w1201, "SlotId"=w1200, "Wavelength Idx"=w1190, "error in (no error)"=w1197, "Intensity"=w1192) -> ("error out"=w1187:errorcluster)  [unwired: 1 in, 1 out]
                n521 = Format Into String(format string="%1$4s OperModeIdx   =>        %2$1d\\r\\n%1$4s WavelengthIdx =>        %3$1d\\r\\n%1$4s Intensity     =>      %4$5.1f %%\\r\\n", initial string="", error in=w1187, w1188, w1189, w1190, w1191) -> (resulting string=w1195:string, error out=w1186:errorcluster)
              }
            }
          }
        }
        n522 = Concatenate Strings(w1047, w1044) -> (w1046:string)
      }
      n523 = local read "cDisplay"() -> (w1043:string)
      n524 = Concatenate Strings(w1043, w1029, w1029, "data values as sent to the device:", w1029, w1029, w1028) -> (w1042:string)
      n525 = local write "cDisplay"(w1042) -> ()
    }
    frame #6 {
      n526 = case shown="No Error" w1205 {
        tunnel: w1204 -> [_ w1212]
        tunnel: w1203 -> [w1207 w1211]
        tunnel: [w1207 w1209] -> w1202
        frame Error {
        }
        frame No Error {
          n527 = Close File(refnum=w1212, error in=w1211) -> (path=w1208:path, error out=w1210:errorcluster)
          n528 = Delete(path (use dialog)=w1208, error in=w1210) -> (error out=w1209:errorcluster)  [unwired: 3 in, 2 out]
        }
      }
    }
    frame #7 {
      n529 = local read "SOMD_NewBurstValues"() -> (→"SOMD_NewBurstValues":T1)
      n530 = local read "VUV_NewTriggerLevel"() -> (→"VUV_NewTriggerLevel":i32)
      n531 = local read "VUV_NewFanRunning"() -> (→"VUV_NewFanRunning":bool)
      n532 = local read "PRI_NewOpModeIdx"() -> (→"PRI_NewOpModeIdx":i32)
      n533 = local read "VUV_NewFreqDivIdx"() -> (→"VUV_NewFreqDivIdx":i32)
      n534 = local read "VUV_NewTrigSrcIdx"() -> (→"VUV_NewTrigSrcIdx":i32)
      n535 = local read "VUV_NewIntensity"() -> (→"VUV_NewIntensity":i32)
      n536 = local read "PRI_NewIntensity"() -> (→"PRI_NewIntensity":u16)
      n537 = local read "PRI_NewWLIdx"() -> (→"PRI_NewWLIdx":i32)
      n538 = local read "SOM_NewBurstLengthArray"() -> (→"SOM_NewBurstLengthArray":i32[])
      n539 = local read "SOM_NewOutNSyncEnable"() -> (→"SOM_NewOutNSyncEnable":T2)
      n540 = local read "SLM_NewPulseParameters"() -> (→"SLM_NewPulseParameters":cluster{"Freq":i32, "PulseMode":u8})
      n541 = local read "SOM_NewFreqTrigMode"() -> (→"SOM_NewFreqTrigMode":i32)
      n542 = local read "SOM_NewBurstValues"() -> (→"SOM_NewBurstValues":T3)
      n543 = local read "VIR_NewTriggerLevel"() -> (→"VIR_NewTriggerLevel":i32)
      n544 = local read "VIR_NewFanRunning"() -> (→"VIR_NewFanRunning":bool)
      n545 = local read "VIR_NewFreqDivIdx"() -> (→"VIR_NewFreqDivIdx":i32)
      n546 = local read "VIR_NewTrigSrcIdx"() -> (→"VIR_NewTrigSrcIdx":i32)
      n547 = local read "SLM_NewIntensity"() -> (→"SLM_NewIntensity":u16)
      n548 = local read "VIR_NewIntensity"() -> (→"VIR_NewIntensity":i32)
      n549 = local read "ModTypFound"() -> (→"ModTypFound":T8)
      n550 = local read "iModuleCount"() -> (→"iModuleCount":i32)
      n551 = local read "SlotNrsFound"() -> (→"SlotNrsFound":T6)
      n552 = local read "SerNrsFound"() -> (→"SerNrsFound":T7)
      n553 = call "FWR Free Module Map.vi"("error in (no error)"=w1213, "DevIdx"=w1214) -> ("error out"=w1215:errorcluster)  [unwired: 1 out]
      n554 = call "USB Close Device.vi"("error in (no error)"=w1215, "DevIdx"=w1214) -> ("error out"=→"error out":errorcluster)
    }
  }
